vi "Process.vi"(8 "error in":errorcluster, 11 "Instrument.DAQ":refnum<class "Instrument.DAQ.lvclass">) -> (0 "error out":errorcluster, 3 "Instrument.DAQ out":refnum<class "Instrument.DAQ.lvclass">)   [LabVIEW 2019, in "Instrument.Lockin.lvlib" / "Instrument.DAQ.lvclass"]
doc: "---------------------------------------------------------------\nJKI State Machine Objects™\nhttp://jki.net/state-machine-objects/\nCopyright (C) 2005-2015, JKI <info@jki.net>\nALL RIGHTS RESERVED"
uses:
  Instrument.DAQ.lvclass
  C:/Program Files/National Instruments/LabVIEW 2019/vi.lib/JKI/JKI SMO/SMO/SMO.lvclass
  Typedefs/Status--enum.ctl
  Typedefs/DAQ.Config.AO.Range--enum.ctl
  Typedefs/DAQ.Type--enum.ctl
  Typedefs/DAQ.Config.AI.Coupling--enum.ctl
  Typedefs/DAQ.Config.AI.Range--enum.ctl
  DAQmx/typedefs/DAQmx.Status--enum.ctl
  Instrument.DAQ.lvclass/Instrument.DAQ.ctl
  Typedefs/Channel.Gain--Cluster.ctl
  Generator/typedefs/Generator.Sweep Status--enum.ctl
  Typedefs/PublicEvents--DAQ.getSweepWaveforms.ctl
  Typedefs/Results--Cluster.ctl
  <vilib>/JKI/JKI SMO/SMO/SMO.lvclass/SMO.ctl
  Typedefs/PrivateEvents--DAQ.setCalibration.ctl
  support/Simulate/Waveguide Model--Cluster.ctl
  Typedefs/PublicEvents--DAQ.getWaveforms.ctl
  Generator/typedefs/Generator.Command--enum.ctl
  6518129d-eb05-4862-8e0f-948d46b99fe2.vi
  19e91f76-1afa-420f-8f76-37c2ee2699b4.vi
  <vilib>/JKI/JKI SMO/SMO/Private/ReftoDVR--SMO.vi
  <vilib>/dlg_ctls.llb/Space Constant.vi
  <vilib>/AdvancedString/1D String Array to Delimited String.vi
  <vilib>/measure/madcrms.llb/Basic Averaged DC-RMS for N Chan.vi
  <vilib>/JKI/JKI SMO/SMO/SMO.lvclass
  <vilib>/measure/NI_MAPro.lvlib
  Instrument.Lockin/Instrument.Lockin.lvclass
  <userlib>/LevyLab/Debug/Debug.lvlib
  DAQmx/DAQmx.lvclass
  DSP/DSP.lvclass
  Waveform.Attributes/Waveform.Attributes.lvlib
  Generator/Generator.lvclass
panel:
  in  "Tab Control":enum32{"Default", "Advanced"}(tab)
  out "Sweep Chart":dbl(graph)
  out "Generator Chart":u32(graph)
  out "DSP Chart":dbl(graph)
  out "Total Chart":dbl(graph)
  out "sweep status":string
  out "Sweep Start":dbl format="%<%.3X>T"
  out "Status":T1=enum."created"
  in  "Calibrate Phase":bool
  in  "Reset Phase":bool
  out "Total (s)":dbl format="%06_6p"
  in  "Auto Phase":bool
  in  "Zero Offset":bool
  in  "Measure Offset":bool
  out "s.h.":string caption="State History"
  out "Payload":variant
  out "Generate (ms)":u32
  out "DSP (s)":dbl format="%0#6_6p"
  in  "Reset REF":bool
  out "Method":string
  out "DAQmx Status":T2
  out "start sweep":string
  out "reset":string
  in  "DAQ AO":T5(array[cluster]) {"configuration" items=["Default"=-1, "Differential"=10106, "Pseudodifferential"=12529]}
  in  "DAQ AI":T8(array[cluster]) {"configuration" items=["default"=-1, "Differential"=10106, "Pseudodifferential"=12529]; "Coupling" items=[""=0, "AC"=10045, "DC"=10050, "GND"=10066]}
  # "For instructions on how to use the JKI State Machine Objects, examples and video tutorials, visit:\nhttp://jki.net/state-machine-objects/\n\nJKI State Machine Objects™\nhttp://jki.net/state-machine-objects/\nCopyright (C) 2005-2015, JKI <info@jki.net>\nALL RIGHTS RESERVED"
  # "DAQ"
  # "State"
  # "Messages"
  # "Sweep"
  # "Controls"
  # "Timing"
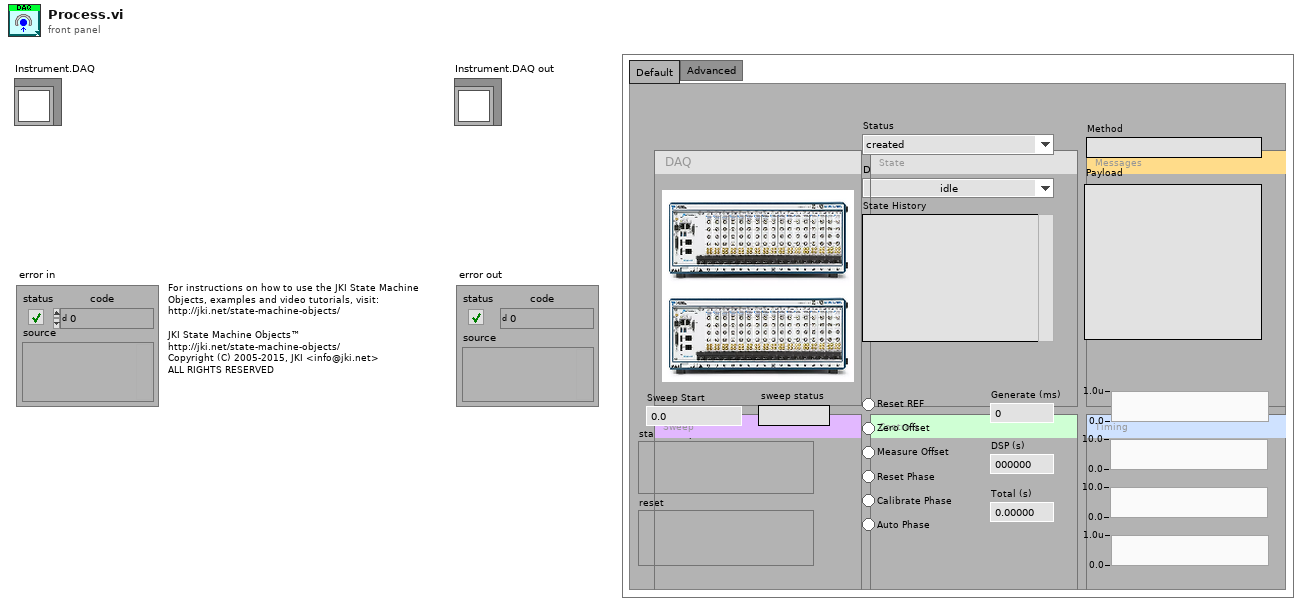
[diagram p1: front panel]
types:
  T1 = typedef "Instrument.Lockin.lvlib/Instrument.DAQ.lvclass/Status--enum.ctl" = enum16{"idle", "created", "started", "stopped", "sweeping"}
  T2 = typedef "DAQmx.lvclass/DAQmx.Status--enum.ctl" = enum16{"idle", "calibrating", "configuring", "creating", "created", "starting", "started", "stopping", "stopped", "clearing", "error"}
  T3 = typedef "Instrument.Lockin.lvlib/Instrument.DAQ.lvclass/DAQ.Config.AO.Range--enum.ctl" = enum16{"±0.1", "±1.0", "±3.5", "±10.0", ""}
  T4 = typedef "Instrument.Lockin.lvlib/Instrument.DAQ.lvclass/DAQ.Type--enum.ctl" = enum16{"None", "USB-4431", "PXI-446x"}
  T5 = cluster{"Channel":tag, "Range":T3, "configuration":i32, "Type":T4}[]
  T6 = typedef "Instrument.Lockin.lvlib/Instrument.DAQ.lvclass/DAQ.Config.AI.Coupling--enum.ctl" = u16
  T7 = typedef "Instrument.Lockin.lvlib/Instrument.DAQ.lvclass/DAQ.Config.AI.Range--enum.ctl" = enum16{"±0.316", "±1.00", "±3.16", "±10.0", "±31.6", "±42.4", ""}
  T8 = cluster{"Channel":tag, "Coupling":T6, "Range":T7, "configuration":i32, "Type":T4}[]
  T9 = typedef "Instrument.Lockin.lvlib/Instrument.DAQ.lvclass/Channel.Gain--Cluster.ctl" = cluster{"Channel":string, "Gain":dbl}
  T10 = enum32{"invalid app kind", "Development System", "Run Time System", "Student Edition", "Embedded LabVIEW", "Evaluation", "Custom"}
  T11 = typedef "Instrument.Lockin.lvlib/Instrument.DAQ.lvclass/PublicEvents--DAQ.getSweepWaveforms.ctl" = cluster{"AO":waveform(dbl)[], "AI":waveform(dbl)[], "X":waveform(dbl)[], "Y":waveform(dbl)[]}
  T12 = enum32{"Invalid", "Standard", "Closed", "Hidden", "Minimized", "Maximized"}
  T13 = typedef "Generator.lvclass/Generator.Sweep Status--enum.ctl" = enum16{"idle", "initializing", "waiting", "sweeping", "stopping"}
  T14 = typedef "Instrument.Lockin.lvlib/Instrument.DAQ.lvclass/PrivateEvents--DAQ.setCalibration.ctl" = enum16{"Check", "Calibrate"}
  T15 = typedef "Instrument.Lockin.lvlib/Instrument.DAQ.lvclass/Waveguide Model--Cluster.ctl" = cluster{"I+":i32, "I-":i32, "V+":i32, "V-":i32, "Vsg":i32}
  T16 = typedef "Instrument.Lockin.lvlib/Instrument.DAQ.lvclass/PublicEvents--DAQ.getWaveforms.ctl" = cluster{"AO":waveform(dbl)[], "AI":waveform(dbl)[], "REF_X":waveform(dbl)[], "REF_Y":waveform(dbl)[], "X":waveform(dbl)[], "Y":waveform(dbl)[]}
  T17 = typedef "Generator.lvclass/Generator.Command--enum.ctl" = enum16{"start", "stop", "start sweep", "stop sweep"}
  T18 = typedef "Instrument.Lockin.lvlib/Instrument.DAQ.lvclass/Results--Cluster.ctl" = cluster{"Time Stamp":timestamp, "Results (Dictionary)":cluster{"key":string, "value":dbl[]}[]}
  T19 = cluster{"Core":cluster{"Current VI Reference":refnum<vi>, "Close Panel on Exit?":bool, "Last Error":cluster{"error":errorcluster, "previous state":string, "remaining states":string}, "Shutdown?":bool}, "SMO":refnum<class "Instrument.DAQ.lvclass">, "DAQ Status":T1, "DAQmx Status":T2, "Sweep Status":T13, "Results":T18, "SweepWaveforms":T11, "Measure Offset":bool, "Saved Amplitudes":dbl[]}
  T20 = typedef "Instrument.Lockin.lvlib/Instrument.DAQ.lvclass/DAQ.Config.AO--Cluster--Array.ctl" = cluster{"Channels":tag, "Range":T3, "terminal configuration":T21, "Type":T4}[]
  T21 = typedef "Instrument.Lockin.lvlib/Instrument.DAQ.lvclass/DAQ.TerminalConfiguration--ring.ctl" = i32
  T22 = cluster{"Channels":tag, "Range":T3, "terminal configuration":T21, "Type":T4}
  T23 = typedef "Instrument.Lockin.lvlib/Instrument.DAQ.lvclass/DAQ.Config.AI--Cluster--Array.ctl" = cluster{"Channels":tag, "Coupling":T6, "Range":T7, "terminal configuration":T21, "Type":T4}[]
  T24 = typedef "Instrument.Lockin.lvlib/Instrument.DAQ.lvclass/Simulation Mode--enum.ctl" = enum16{"AI = HW simulated", "AI = noise*AO", "AI = waveguide"}
  T25 = cluster{"AI Configuration":T23, "Simulation mode":T24}
  T26 = cluster{"Channels":tag, "Coupling":T6, "Range":T7, "terminal configuration":T21, "Type":T4}
  T27 = typedef "Instrument.Lockin.lvlib/Instrument.DAQ.lvclass/AO.Channel--Cluster--Array.ctl" = T28[]
  T28 = typedef "Instrument.Lockin.lvlib/Instrument.DAQ.lvclass/AO.Channel--Cluster.ctl" = cluster{"Enable?":bool, "Channel":i32, "Amplitude":dbl, "Offset":dbl, "Frequency":dbl, "Phase":dbl, "Function":T29, "Sweeping?":bool, "Limit AC":bool, "Limit DC?":bool, "Duty Cycle":bool}
  T29 = typedef "Instrument.Lockin.lvlib/Instrument.DAQ.lvclass/AO.Channel.Function--Enum.ctl" = enum16{"sine", "square", "triangle", "saw"}
  T30 = typedef "Instrument.Lockin.lvlib/Instrument.DAQ.lvclass/AI.Channel--Cluster--Array.ctl" = T31[]
  T31 = typedef "Instrument.Lockin.lvlib/Instrument.DAQ.lvclass/AI.Channel--Cluster.ctl" = cluster{"Enable?":bool, "Channel":i32, "References":u16[], "reference index":i32}
  T32 = typedef "Instrument.Lockin.lvlib/Instrument.DAQ.lvclass/REF.Channel--Cluster--Array.ctl" = T33[]
  T33 = typedef "Instrument.Lockin.lvlib/Instrument.DAQ.lvclass/REF.Channel--Cluster.ctl" = cluster{"Enable?":bool, "Channel":i32, "Frequency":dbl, "Phase":dbl, "TC":dbl, "Roll-Off":i32}
  T34 = typedef "Instrument.Lockin.lvlib/Instrument.DAQ.lvclass/DAQ.Sampling--Cluster.ctl" = cluster{"Sampling":T35, "sample mode":i32, "Fs Mode":T36, "Fs Multiplier":dbl, "Refresh Rate (Hz)":dbl, "Decimation.PreDSP":i32, "Decimation.PostDSP":i32, "Fs.Output":dbl}
  T35 = typedef "Instrument.Lockin.lvlib/Instrument.DAQ.lvclass/DAQ.Sampling.Sampling--Cluster.ctl" = cluster{"Fs":dbl, "#s":i32}
  T36 = typedef "Instrument.Lockin.lvlib/Instrument.DAQ.lvclass/DAQ.Sampling.Fs Mode--enum.ctl" = enum16{"Manual", "Auto Fs", "Max Fs"}
  T37 = typedef "Instrument.Lockin.lvlib/Instrument.DAQ.lvclass/Sweep.Configuration--Cluster.ctl" = cluster{"sweepTime":dbl, "initialWaitTime":dbl, "returnToStart":bool, "sweepChannels":T38}
  T38 = typedef "Instrument.Lockin.lvlib/Instrument.DAQ.lvclass/Sweep.Channel--Cluster--Array.ctl" = T39[]
  T39 = typedef "Instrument.Lockin.lvlib/Instrument.DAQ.lvclass/Sweep.Channel--Cluster.ctl" = cluster{"Enable?":bool, "Channel":u16, "Start":dbl, "End":dbl, "Pattern":T40, "Table":dbl[]}
  T40 = typedef "Instrument.Lockin.lvlib/Instrument.DAQ.lvclass/Sweep.Pattern--Enum.ctl" = enum16{"Ramp /", "Ramp /\\", "Smooth Ramp _/", "Smooth Ramp _/\\_", "Table"}
  T41 = typedef "Instrument.Lockin.lvlib/Instrument.DAQ.lvclass/PrivateEvents--DAQ.measureOffset.ctl" = bool
  T42 = typedef "Instrument.Lockin.lvlib/Instrument.DAQ.lvclass/PrivateEvents--DAQ.zeroPhase.ctl" = bool
  T43 = typedef "Instrument.Lockin.lvlib/Instrument.DAQ.lvclass/Configuration.Prefilter--Cluster.ctl" = cluster{"60 Hz":bool, "Low Pass":bool, "Low Pass Cutoff (Hz)":dbl}
  T44 = typedef "Instrument.Lockin.lvlib/Instrument.DAQ.lvclass/Configuration.AmplitudeLimit--Cluster.ctl" = cluster{"Limit?":bool, "Limit (V)":dbl}
  T45 = typedef "Instrument.Lockin.lvlib/Instrument.DAQ.lvclass/Configuration.DCLimit--Cluster.ctl" = cluster{"Limit?":bool, "Limit (V)":dbl}
  T46 = typedef "Instrument.Lockin.lvlib/Instrument.DAQ.lvclass/Configuration.DutyCycle--Cluster.ctl" = cluster{"Option?":bool, "Duty Cycle (%)":dbl}
  T47 = typedef "Instrument.Lockin.lvlib/Instrument.DAQ.lvclass/Configuration.LinkFrequencies--Cluster.ctl" = cluster{"Link?":bool, "Frequency (Hz)":dbl}
  T48 = typedef "Instrument.Lockin.lvlib/Instrument.DAQ.lvclass/State--enum.ctl" = enum16{"start", "stop", "reset", "start sweep", "stop sweep"}
  T49 = typedef "Instrument.Lockin.lvlib/Instrument.DAQ.lvclass/PrivateEvents--DAQ.showUI.ctl" = bool
  T50 = typedef "DAQmx.lvclass/DeviceInfo--Cluster.ctl" = cluster{"DeviceName":string, "DevIsSimulated":bool, "DeviceSerialNumber":string, "ProductType":string, "ProductCategory":i32, "ProductNumber":u32, "ChassisNumber":u32, "SlotNumber":u32, "ChassisName":string, "ChassisSerialNumber":string, "DevTemp":dbl, "SelfCal.LastDate/Time":string, "SelfCal.LastTemp":dbl, "calibration due?":bool}
  T51 = cluster{"Active Device":string, "SelfCal.LastDate/Time":string, "SelfCal.LastTemp":dbl, "DevTemp":dbl, "calibration due?":bool}[]
  T52 = typedef "Instrument.Lockin.lvlib/Instrument.DAQ.lvclass/DAQ.Calibration--Cluster.ctl" = cluster{"Active Device":string, "SelfCal.LastDate/Time":dbl, "SelfCal.LastTemp":dbl, "DevTemp":dbl, "calibration due?":bool}
  T53 = typedef "DAQmx.lvclass/DAQ.Config.AO--Cluster--Array.ctl" = T54[]
  T54 = typedef "DAQmx.lvclass/DAQ.Config.AO--Cluster.ctl" = cluster{"Channels":tag, "Range":T55, "output terminal configuration":i32, "Type":T56}
  T55 = typedef "DAQmx.lvclass/DAQ.Config.AO.Range--enum.ctl" = enum16{"±0.1", "±1.0", "±3.5", "±10.0", ""}
  T56 = typedef "DAQmx.lvclass/DAQ.Config.Device Type--enum.ctl" = enum16{"None", "USB-4431", "PXI-446x"}
  T57 = typedef "DAQmx.lvclass/DAQ.Config.AI--Cluster--Array.ctl" = T58[]
  T58 = typedef "DAQmx.lvclass/DAQ.Config.AI--Cluster.ctl" = cluster{"Channels":tag, "Coupling":T59, "Range":T60, "input terminal configuration":i32, "Type":T56}
  T59 = typedef "DAQmx.lvclass/DAQ.Config.AI.Coupling--enum.ctl" = u16
  T60 = typedef "DAQmx.lvclass/DAQ.Config.AI.Range--enum.ctl" = enum16{"±0.316", "±1.00", "±3.16", "±10.0", "±31.6", "±42.4", ""}
  T61 = typedef "Generator.lvclass/AO.Channel--Cluster--Array.ctl" = T62[]
  T62 = typedef "Generator.lvclass/AO.Channel--Cluster.ctl" = cluster{"Enable?":bool, "Channel":i32, "Amplitude":dbl, "Offset":dbl, "Frequency":dbl, "Phase":dbl, "Function":T63, "Sweeping?":bool, "Limit AC?":bool, "Limit DC?":bool, "Duty Cycle?":bool, "Duty Cycle":dbl}
  T63 = typedef "Generator.lvclass/AO.Channel.Function--Enum.ctl" = enum16{"sine", "square", "triangle", "saw"}
  T64 = cluster{"Current VI Reference":refnum<vi>, "Close Panel on Exit?":bool, "Last Error":cluster{"error":errorcluster, "previous state":string, "remaining states":string}, "Shutdown?":bool}
  T65 = typedef "Instrument.Lockin.lvlib/Instrument.DAQ.lvclass/DeviceInfo--Cluster.ctl" = cluster{"DeviceName":string, "DevIsSimulated":bool, "DeviceSerialNumber":string, "ProductType":string, "ProductCategory":i32, "ProductNumber":u32, "ChassisNumber":u32, "SlotNumber":u32, "ChassisName":string, "ChassisSerialNumber":string, "DevTemp":dbl, "SelfCal.LastDate/Time":string, "SelfCal.LastTemp":dbl, "calibration due?":bool}
  T66 = typedef "Instrument.Lockin.lvlib/Instrument.DAQ.lvclass/DAQ.Calibration--Cluster--Array.ctl" = T52[]
  T67 = typedef "Instrument.Lockin.lvlib/Instrument.DAQ.lvclass/DAQ.Configuration--Cluster--Array.ctl" = T68[]
  T68 = typedef "Instrument.Lockin.lvlib/Instrument.DAQ.lvclass/DAQ.Configuration--Cluster.ctl" = cluster{"Device":string, "Lockin.AO":string, "AO.Ch":string, "AO.Range":T3, "AO terminal config":T21, "Lockin.AI":string, "AI.Ch":string, "AI.Range":T7, "AI.Coupling":T6, "AI terminal config":T21}
  T69 = typedef "Instrument.Lockin.lvlib/Instrument.DAQ.lvclass/Channel.Gain--Cluster--Array.ctl" = T9[]
  T70 = typedef "Debug.lvlib/Attribute.Debug.lvclass/DebugBehavior.ctl" = enum16{"Normal", "Debug"}
  T71 = typedef "SMO.lvclass/Protected Events.ctl" = cluster{"StopProcesses":refnum<user-event>, "AbortProcesses":refnum<user-event>, "Config Changed":refnum<user-event>, "Dependency":refnum<user-event>}
  T72 = typedef "Instrument.Lockin.lvlib/Instrument.DAQ.lvclass/PrivateEvents--Cluster.ctl" = cluster{"setAOconfig":refnum<user-event>, "setAIconfig":refnum<user-event>, "setAO":refnum<user-event>, "setREF":refnum<user-event>, "setSampling":refnum<user-event>, "setState":refnum<user-event>, "setInputGain":refnum<user-event>, "setOutputGain":refnum<user-event>, "setSweep":refnum<user-event>, "measureOffset":refnum<user-event>, "zeroOffset":refnum<user-event>, "setPreFilter":refnum<user-event>, "autoConfigureDAQ":refnum<user-event>, "setCalibration":refnum<user-event>, "setAI":refnum<user-event>, "zeroPhase":refnum<user-event>, "setAmplitudeLimit":refnum<user-event>, "setLinkFrequencies":refnum<user-event>, "showUI":refnum<user-event>, "setInputOffset":refnum<user-event>, "setDCLimit":refnum<user-event>, "setDutyCycle":refnum<user-event>}
  T73 = typedef "DAQmx.lvclass/PublicEvents--Cluster.ctl" = cluster{"Status":refnum<user-event>, "Devices":refnum<user-event>, "Calibration":refnum<user-event>, "Sampling":refnum<user-event>, "AOconfig":refnum<user-event>, "AIconfig":refnum<user-event>, "Waveforms":refnum<user-event>}
  T74 = typedef "Generator.lvclass/PublicEvents--Cluster.ctl" = cluster{"Status":refnum<user-event>, "SweepStatus":refnum<user-event>, "AOChannels":refnum<user-event>, "Waveforms":refnum<user-event>}
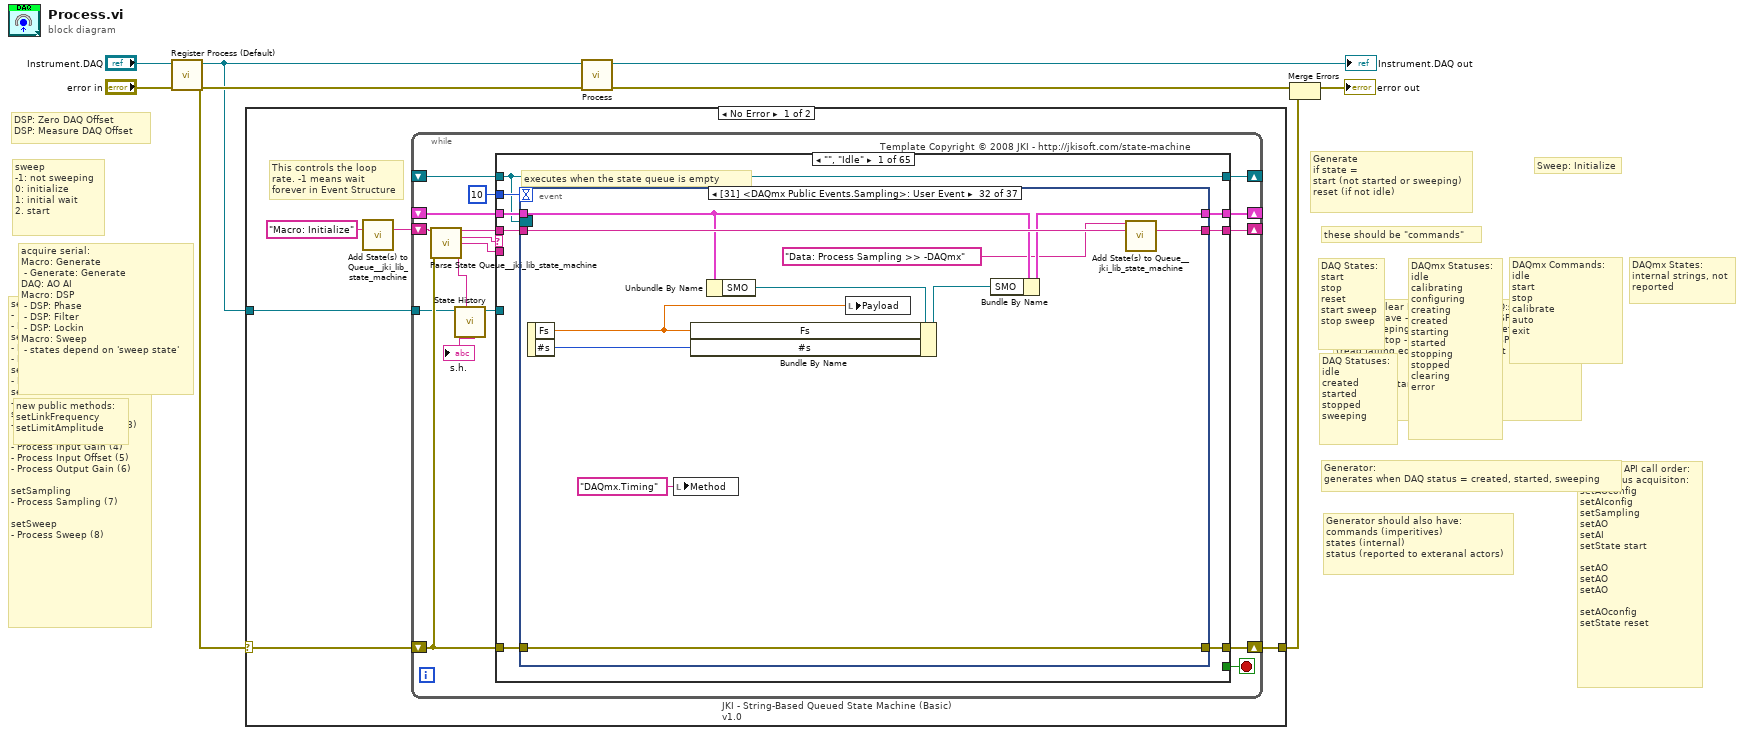
[diagram p0: block diagram]
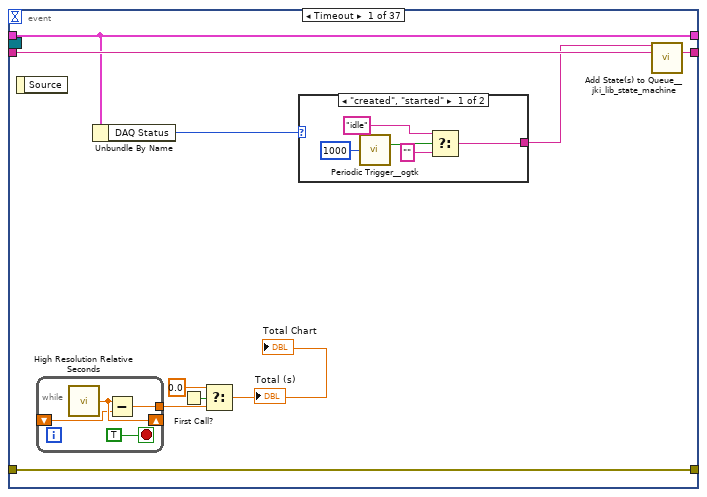
[diagram p2: hidden frame]
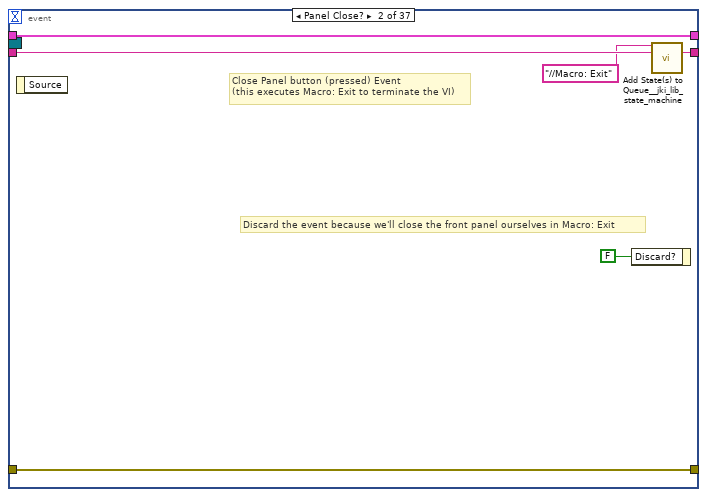
[diagram p4: hidden frame]
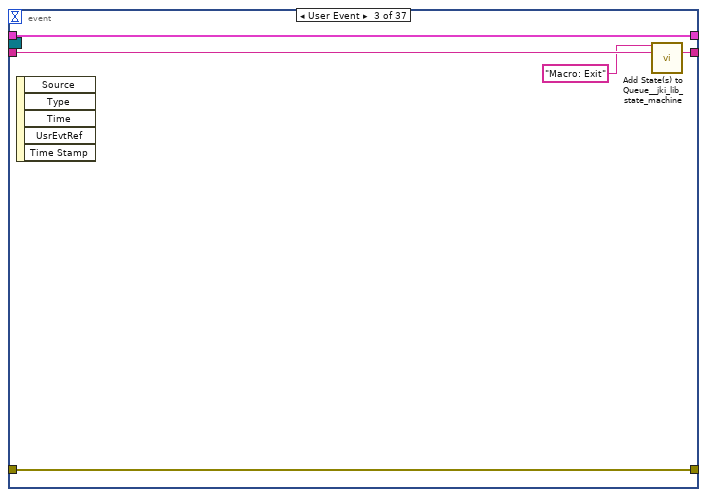
[diagram p5: hidden frame]
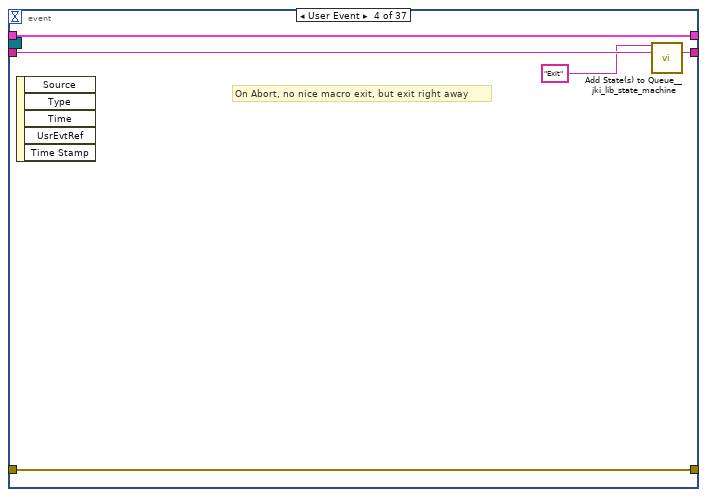
[diagram p6: hidden frame]
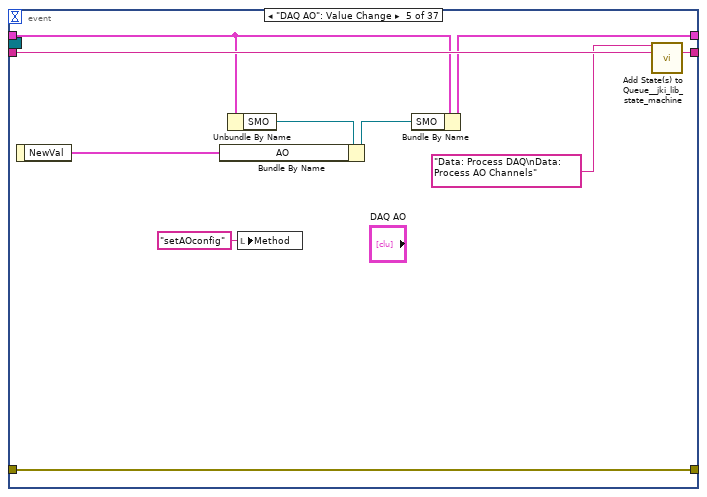
[diagram p7: hidden frame]
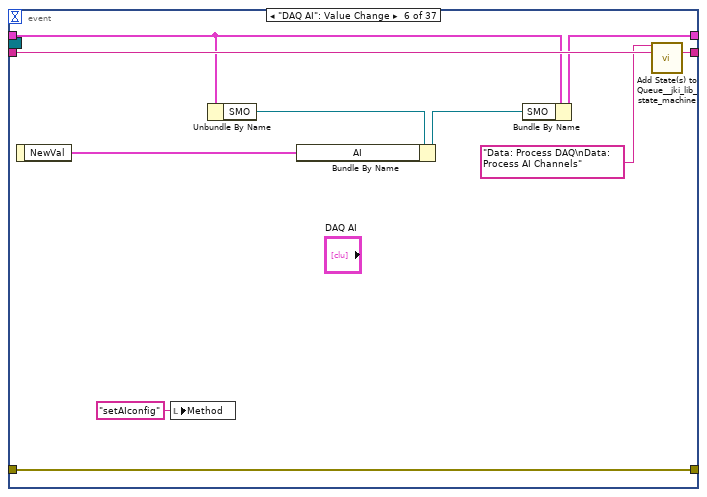
[diagram p8: hidden frame]
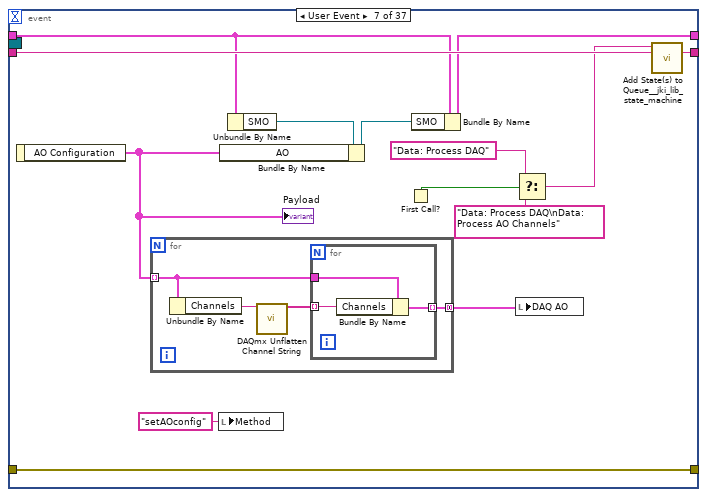
[diagram p9: hidden frame]
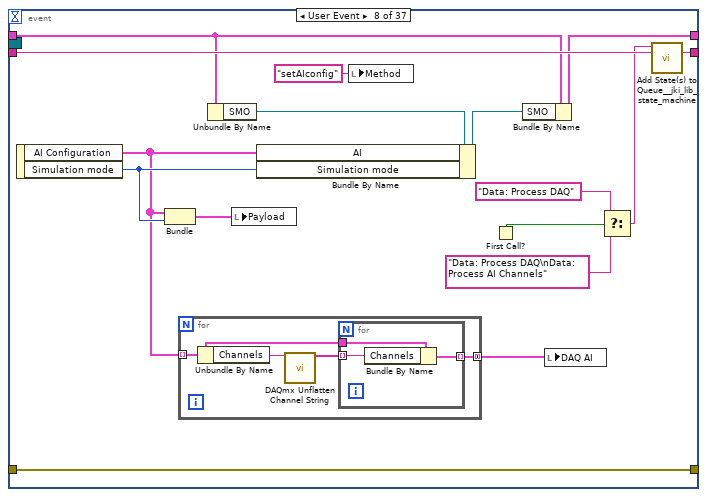
[diagram p10: hidden frame]
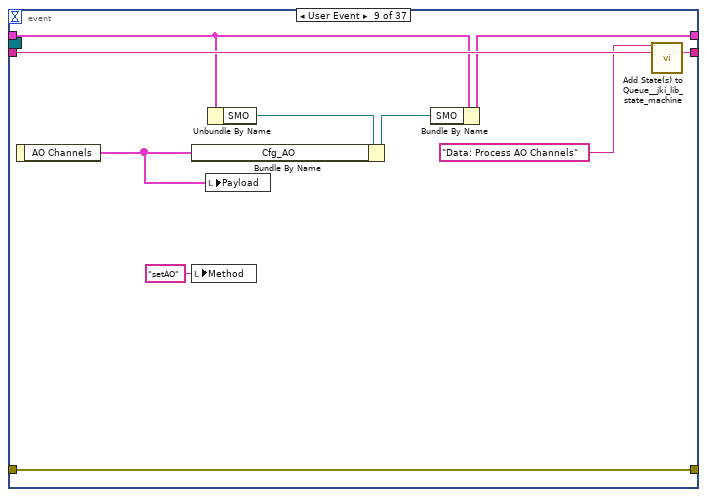
[diagram p11: hidden frame]
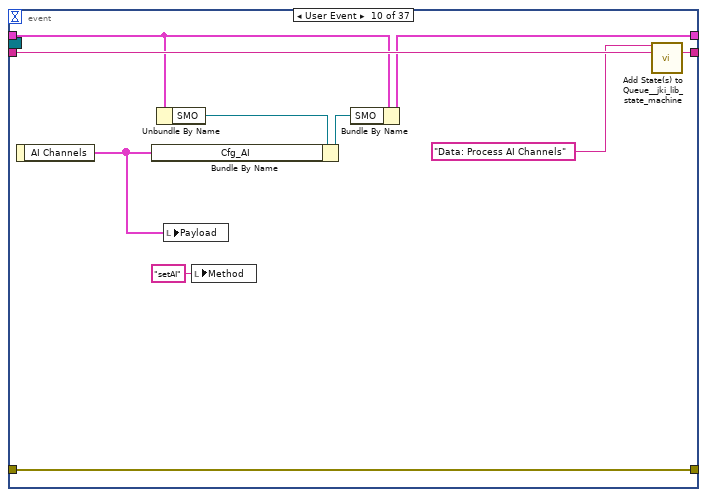
[diagram p12: hidden frame]
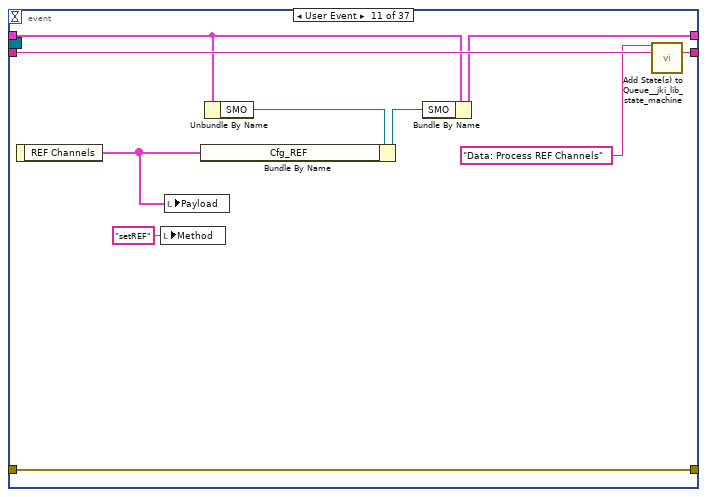
[diagram p13: hidden frame]
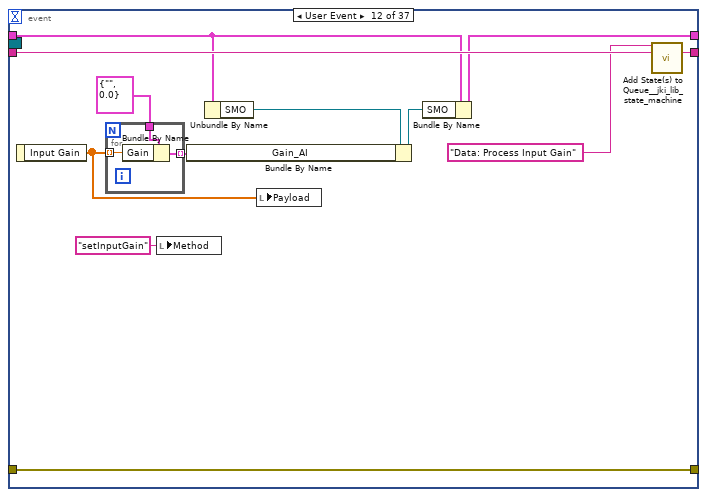
[diagram p14: hidden frame]
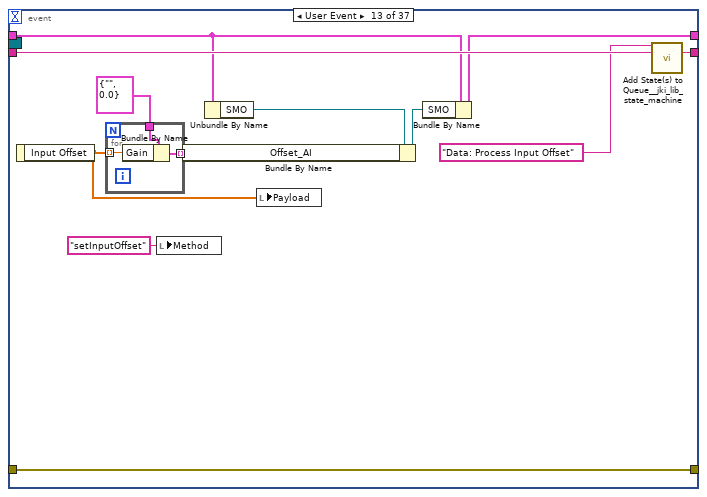
[diagram p15: hidden frame]
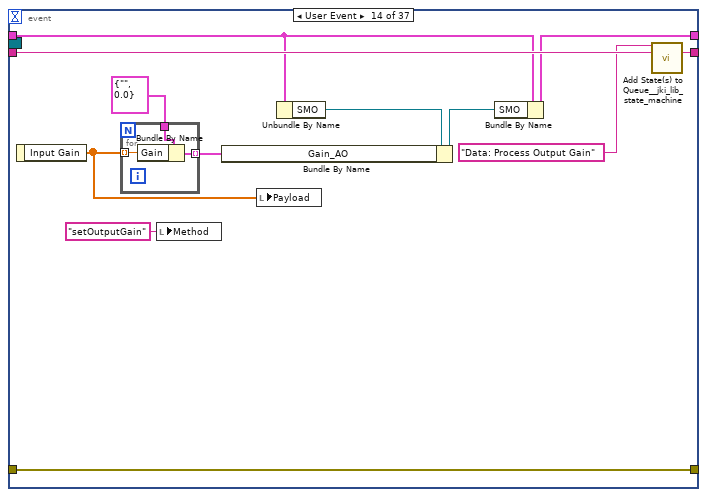
[diagram p16: hidden frame]
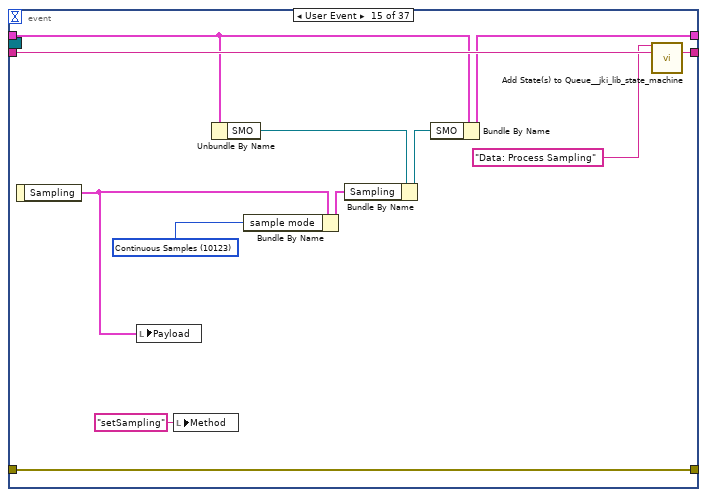
[diagram p17: hidden frame]
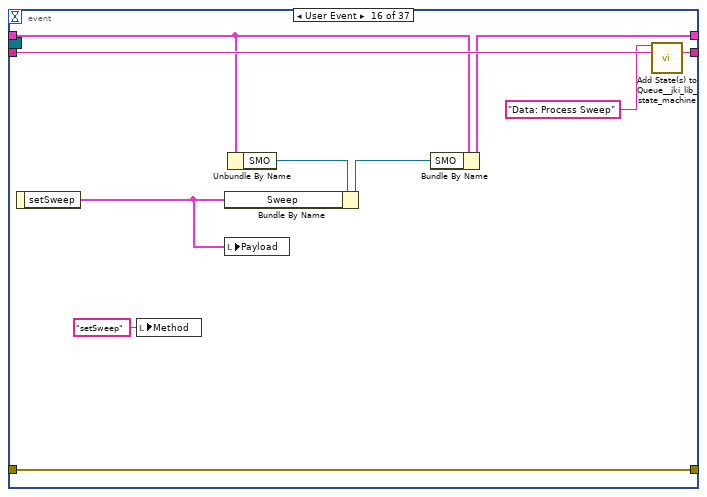
[diagram p18: hidden frame]
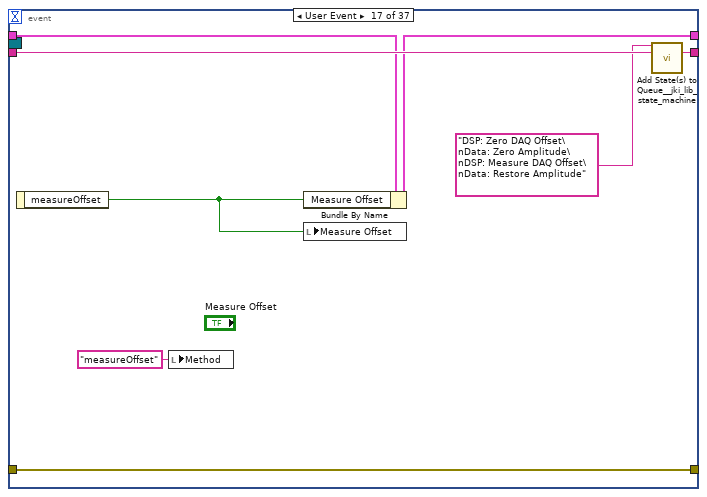
[diagram p19: hidden frame]
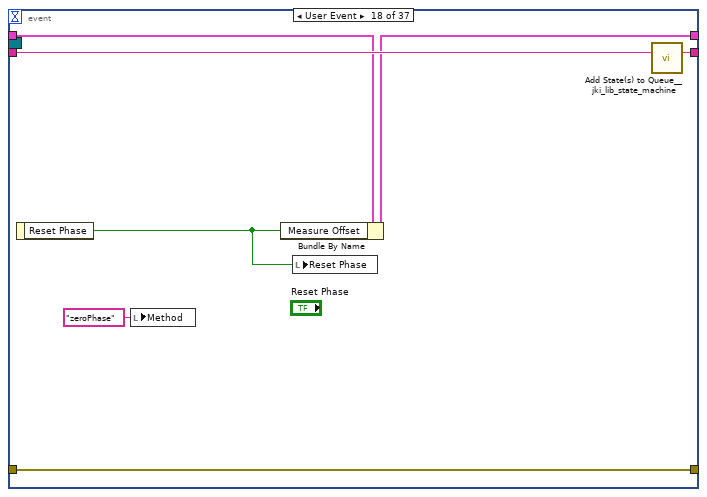
[diagram p20: hidden frame]
diagram:
  # "Sweep: Initialize"
  # "- Sweep: Clear Data - called by DAQ:setState\n- Sweep: Save - called by Macro: DSP\n(read sweeping attribute from waveform)\n- Sweep: Stop - called by Macro: DSP\n(read falling edge sweeping --> not sweeping)\n\n\nGenerator: Start, Stop"
  # "example API call order:\ncontinuous acquisiton:\nsetAOconfig\nsetAIconfig\nsetSampling\nsetAO\nsetAI\nsetState start\n\nsetAO\nsetAO\nsetAO\n\nsetAOconfig\nsetState reset"
  # "Generator should also have:\ncommands (imperitives)\nstates (internal)\nstatus (reported to exteranal actors)"
  # "these should be \"commands\""
  # "DAQmx States:\ninternal strings, not\nreported"
  # "DAQmx Commands:\nidle\nstart\nstop\ncalibrate\nauto\nexit"
  # "Generator:\ngenerates when DAQ status = created, started, sweeping"
  # "DAQmx Statuses:\nidle\ncalibrating\nconfiguring\ncreating\ncreated\nstarting\nstarted\nstopping\nstopped\nclearing\nerror"
  # "DAQ Statuses:\nidle\ncreated\nstarted\nstopped\nsweeping"
  # "DAQ States:\nstart\nstop\nreset\nstart sweep\nstop sweep"
  # "Generate\nif state = \nstart (not started or sweeping)\nreset (if not idle)"
  # "setAOconfig:\n-\t Process DAQ (0)\n- Process AO Channels (1)\nsetAOconfig\n- Process DAQ\n- Process AI Channels (2)\nsetAO\n- Process AO Channels\nsetAI\n- Process AI Channels\nsetREF\n- Process REF Channels (3)\n\n- Process Input Gain (4)\n- Process Input Offset (5)\n- Process Output Gain (6)\n\nsetSampling\n- Process Sampling (7)\n\nsetSweep\n- Process Sweep (8)"
  # "acquire serial:\nMacro: Generate\n - Generate: Generate\nDAQ: AO AI\nMacro: DSP\n - DSP: Phase\n - DSP: Filter\n - DSP: Lockin\nMacro: Sweep\n - states depend on 'sweep state'"
  # "sweep\n-1: not sweeping\n0: initialize\n1: initial wait\n2. start"
  # "DSP: Zero DAQ Offset\nDSP: Measure DAQ Offset"
  # "new public methods:\nsetLinkFrequency\nsetLimitAmplitude"
  n1 = call <vilib>:"Register Process (Default).vi"("error in (no error)"="error in", "SMO"="Instrument.DAQ") -> ("error out"=w5:errorcluster, "SelfRef"=w4:refnum<class "Instrument.DAQ.lvclass">)  [unwired: 8 in]
  n2 = case shown="No Error" w5 {
    selector: w5 -> [w13 w1355]
    tunnel: w4 -> [w9 _]
    tunnel: [w12 w1355] -> w1
    frame No Error {
      # "This controls the loop rate. -1 means wait forever in Event Structure"
      n3 = call <vilib>:"Add State(s) to Queue__jki_lib_state_machine.vi"("State(s) in (\"\")"="Macro: Initialize") -> ("States Out"=w11:string)  [unwired: 14 in]
      n4 = while "JKI - String-Based Queued State Machine (Basic) v1.0" {
        shift-right: [w24] -> _
        shift-left: _ -> [w20]
        shift-right: [w19] -> w12
        shift-left: w13 -> [w23]
        shift-right: [w26] -> _
        shift-left: w11 -> [w27]
        tunnel: w9 -> [w14]
        shift-right: [w22] -> _
        shift-left: _ -> [w21]
        stop <- w25 stop-if-true
        # "Template Copyright © 2008 JKI - http://jkisoft.com/state-machine"
        n5 = call <vilib>:"Parse State Queue__jki_lib_state_machine.vi"("State Queue"=w27, "Error In (no error)"=w23) -> ("Remaining States"=w29:string, "Current State"=w17:string, "Arguments"=w28:string)  [unwired: 11 in]
        n6 = call <userlib>:"State History.vi"("Current State"=w17, "SMO"=w14) -> ("SMO"=w15:refnum<class "Instrument.DAQ.lvclass">, "History"=→"s.h.":string)  [unwired: 8 in]
        n7 = case shown="\"\", \"Idle\"" w17 {
          selector: w17 -> [_ _ w473 _ _ _ _ _ _ _ _ _ _ _ _ _ _ _ _ _ _ _ _ _ _ _ _ _ _ w867 _ _ _ _ _ _ _ _ _ _ _ _ _ _ _ _ _ _ _ _ _ _ _ _ _ _ _ _ _ _ _ _ _ _ _]
          tunnel: w29 -> [w37 w471 w477 w496 w498 w515 w520 w535 w546 w567 w577 w593 w622 w643 w668 w688 w700 w712 w724 w741 w750 w765 w775 w787 w811 w832 w848 w853 w862 w878 w885 w901 w933 w942 w957 w976 w1010 w1017 w1034 w1064 w1069 w1080 w1085 w1105 w1111 w1116 w1125 w1134 w1147 w1164 w1169 w1179 w1199 w1229 w1246 w1264 w1284 w1301 w1306 w1313 w1318 w1327 w1336 w1345 w1354]
          tunnel: w28 -> [_ _ _ _ _ _ _ _ _ _ _ w578 w615 _ _ _ _ _ _ _ _ _ _ _ w789 _ _ _ _ w863 w879 w895 _ _ _ _ _ _ _ _ _ _ _ _ _ _ _ _ w1136 _ _ _ _ _ _ _ _ _ _ _ _ _ _ _ _]
          tunnel: w20 -> [w35 w468 w475 w487 w507 w511 w517 _ w540 w562 w568 w589 w618 w639 w664 w684 w695 w708 w719 w737 w746 w759 w771 w783 w807 w826 w842 w850 w860 w875 w883 w897 w930 w938 w945 w965 w994 w1012 w1028 w1054 w1066 w1077 w1082 w1103 w1109 w1114 w1120 w1131 w1144 w1161 w1167 w1172 w1195 w1226 w1243 w1260 w1281 w1297 w1304 w1307 w1316 w1324 w1333 w1342 w1351]
          tunnel: w23 -> [w33 w469 w478 w493 w499 _ w518 w528 w541 w559 w570 w582 w608 w636 w662 w683 w691 w702 w714 w735 w742 w757 w769 w781 w798 w828 w845 w851 w856 w876 w881 w899 w931 w940 w943 w974 w1008 w1015 w1033 w1049 w1067 w1072 w1083 w1088 w1108 w1112 w1121 w1126 w1141 w1157 w1165 w1174 w1192 w1223 w1232 w1261 w1266 w1294 w1302 w1310 w1314 w1320 w1329 w1338 w1347]
          tunnel: [w36 w470 w476 w495 w502 w514 w519 w534 w545 w566 w576 w592 w621 w642 w667 w687 w699 w711 w723 w740 w749 w764 w774 w786 w810 w831 w847 w852 w861 w877 w884 w900 w932 w941 w956 w975 w1009 w1016 w1031 w1063 w1068 w1079 w1084 w1104 w1110 w1115 w1124 w1133 w1146 w1163 w1168 w1178 w1198 w1228 w1245 w1263 w1283 w1300 w1305 w1312 w1317 w1326 w1335 w1344 w1353] -> w26
          tunnel: [_ _ _ _ _ TRUE _ _ _ _ _ _ _ _ _ _ _ _ _ _ _ _ _ _ _ _ _ _ _ _ _ _ _ _ _ _ _ _ _ _ _ _ _ _ _ _ _ _ _ _ _ _ _ _ _ _ _ _ _ _ _ _ _ _ _] -> w25
          tunnel: [w32 w468 w475 w494 w506 w511 w517 w532 w542 w563 w569 w590 w619 w640 w665 w685 w696 w709 w720 w738 w746 w760 w772 w784 w808 w827 w842 w850 w860 w875 w883 w897 w930 w938 w947 w966 w995 w1012 w1028 w1054 w1066 w1077 w1082 w1103 w1109 w1114 w1119 w1130 w1143 w1160 w1167 w1173 w1194 w1225 w1242 w1260 w1280 w1296 w1304 w1307 w1316 w1324 w1333 w1342 w1351] -> w24
          tunnel: 10 ("to") -> [w31 _ _ _ _ _ _ _ _ _ _ _ _ _ _ _ _ _ _ _ _ _ _ _ _ _ _ _ _ _ _ _ _ _ _ _ _ _ _ _ _ _ _ _ _ _ _ _ _ _ _ _ _ _ _ _ _ _ _ _ _ _ _ _ _]
          tunnel: w15 -> [_ _ _ _ _ _ _ w527 _ _ _ _ _ _ _ _ _ _ _ _ _ _ _ _ _ _ _ _ _ _ _ _ _ _ _ _ _ _ _ _ _ _ _ _ _ _ _ _ _ _ _ _ _ _ _ _ _ _ _ _ _ _ _ _ _]
          tunnel: [w30 w467 w472 w484 w509 w512 w516 w533 w544 w565 w575 w591 w620 w641 w666 w686 w698 w710 w722 w739 w748 w763 w773 w785 w809 w830 w843 w849 w859 w874 w882 w894 w929 w939 w955 w973 w1003 w1014 w1032 w1062 w1065 w1078 w1081 w1097 w1106 w1113 w1123 w1132 w1145 w1162 w1166 w1177 w1197 w1227 w1244 w1262 w1282 w1299 w1303 w1311 w1315 w1325 w1334 w1343 w1352] -> w22
          tunnel: w21 -> [w30 w467 w472 w484 w509 w512 w516 w533 w544 w565 w575 w591 w620 w641 w666 w686 w698 w710 w722 w739 w748 w763 w773 w785 w809 w830 w843 w849 w859 w874 w882 w894 w929 w939 w955 w973 w1003 w1014 w1032 w1062 w1065 w1078 w1081 _ w1106 w1113 w1123 w1132 w1145 w1162 w1166 w1177 w1197 w1227 w1244 w1262 w1282 w1299 w1303 w1311 w1315 w1325 w1334 w1343 w1352]
          tunnel: [w34 w469 w479 w493 errorcluster {"status"=FALSE, "code"=0, "source"=""} ("No error") w510 w518 w530 w537 w560 w571 w579 w604 w631 w655 w669 w690 w706 w715 w734 w743 w758 w768 w779 w797 w829 w844 w851 w857 w876 w880 w898 w931 w940 w944 w974 w1008 w1015 w1033 w1050 w1067 w1071 w1083 w1101 w1108 w1112 w1117 w1127 w1140 w1156 w1165 w1175 w1185 w1213 w1237 w1261 w1267 w1288 w1302 w1310 w1314 w1321 w1330 w1339 w1348] -> w19
          frame "", "Idle" {
            # "executes when the state queue is empty"
            n8 = event shown="[31] <DAQmx Public Events.Sampling>: User Event" {
              selector: w30 -> [_ _ _ _ _ _ _ _ _ _ _ _ _ _ _ _ _ _ _ _ _ _ _ _ _ _ _ _ _ _ _ _ _ _ _ _ _]
              dyn-events: _ -> [_ _ _ _ _ _ _ _ _ _ _ _ _ _ _ _ _ _ _ _ _ _ _ _ _ _ _ _ _ _ _ _ _ _ _ _ _]
              timeout: w31 -> [_ _ _ _ _ _ _ _ _ _ _ _ _ _ _ _ _ _ _ _ _ _ _ _ _ _ _ _ _ _ _ _ _ _ _ _ _]
              tunnel: w37 -> [w42 w63 w68 w73 w83 w93 w107 w130 w147 w157 w167 w179 w194 w209 w224 w234 w242 w249 w255 w265 w275 w285 w295 w305 w312 w320 w342 w353 w360 w370 w381 w392 w402 w412 w430 w445 w459]
              tunnel: [w47 w62 w67 w72 w82 w92 w106 w129 w146 w156 w166 w178 w193 w208 w223 w233 w241 w248 w254 w264 w274 w284 w294 w304 w311 w319 w341 w352 w361 w371 w382 w393 w403 w413 w431 w444 w460] -> w36
              tunnel: w35 -> [w41 w60 w65 w70 w79 w89 w103 w126 w143 w153 w163 w175 w190 w205 w221 w230 w238 w246 w252 w260 w270 w280 w290 w300 w309 w314 w337 w349 w358 w366 w377 w387 w395 w406 w426 w440 w462]
              tunnel: [w46 w61 w66 w71 w76 w86 w100 w121 w142 w148 w159 w172 w187 w204 w219 w231 w240 w247 w253 w263 w273 w283 w293 w303 w310 w318 w340 w351 w357 w365 w376 w391 w401 w411 w422 w439 w454] -> w34
              tunnel: w33 -> [w46 w61 w66 w71 w76 w86 w100 w121 w142 w148 w159 w172 w187 w204 w219 w231 w240 w247 w253 w263 w273 w283 w293 w303 w310 w318 w340 w351 w357 w365 w376 w391 w401 w411 w421 w438 w461]
              tunnel: [w41 w60 w65 w70 w81 w91 w105 w128 w145 w155 w165 w177 w192 w207 w217 w232 w237 w245 w252 w261 w271 w281 w291 w301 w309 w314 w337 w349 w356 w367 w378 w386 w396 w407 w427 w440 w463] -> w32
              event Timeout {
                n9 = event-data() -> ()  [unwired: 1 in, 1 out]
                n10 = while {
                  shift-right: [w57] -> _
                  shift-left: _ -> [w56]
                  tunnel: [w55] -> w44
                  stop <- TRUE stop-if-true
                  n11 = call <vilib>:"High Resolution Relative Seconds.vi"() -> ("relative seconds"=w57:dbl)
                  n12 = Subtract(x=w57, y=w56) -> (x-y=w55:dbl)
                }
                n13 = Unbundle By Name(w41) -> ("DAQ Status"=w40:T1)
                n14 = First Call?() -> (First Call?: T/F=w43:bool)
                n15 = Select(t=0.0, s=w43, f=w44) -> (s? t:f=→"Total (s)" →"Total Chart":dbl)
                n16 = case shown="\"created\", \"started\"" w40 {
                  tunnel: [w50 "" ("State(s) in Front (\"\")")] -> w39
                  frame "created", "started" {
                    n17 = call <userlib>:"Periodic Trigger__ogtk.vi"("time (ms)"=u32 1000) -> ("Triggered"=w52:bool)  [unwired: 12 in, 2 out]
                    n18 = Select(t="idle" ("State(s) in Front (\"\")"), s=w52, f="") -> (s? t:f=w50:string)
                  }
                  frame "idle", "stopped", "sweeping" {
                  }
                }
                n19 = call <vilib>:"Add State(s) to Queue__jki_lib_state_machine.vi"("State(s) in Front (\"\")"=w39, "State(s) in (\"\")"=w42) -> ("States Out"=w47:string)  [unwired: 13 in]
              }
              event Panel Close? {
                # "Discard the event because we'll close the front panel ourselves in Macro: Exit"
                # "Close Panel button (pressed) Event\n(this executes Macro: Exit to terminate the VI)"
                n20 = event-data() -> ()  [unwired: 1 in, 1 out]
                n21 = event-data("Discard?"=FALSE) -> ()  [unwired: 1 in, 1 out]
                n22 = call <vilib>:"Add State(s) to Queue__jki_lib_state_machine.vi"("State(s) in Front (\"\")"="//Macro: Exit", "State(s) in (\"\")"=w63) -> ("States Out"=w62:string)  [unwired: 13 in]
              }
              event User Event {
                n23 = event-data() -> ()  [unwired: 1 in, 5 out]
                n24 = call <vilib>:"Add State(s) to Queue__jki_lib_state_machine.vi"("State(s) in Front (\"\")"="Macro: Exit", "State(s) in (\"\")"=w68) -> ("States Out"=w67:string)  [unwired: 13 in]
              }
              event User Event {
                # "On Abort, no nice macro exit, but exit right away"
                n25 = event-data() -> ()  [unwired: 1 in, 5 out]
                n26 = call <vilib>:"Add State(s) to Queue__jki_lib_state_machine.vi"("State(s) in Front (\"\")"="Exit", "State(s) in (\"\")"=w73) -> ("States Out"=w72:string)  [unwired: 13 in]
              }
              event "DAQ AO": Value Change {
                n27 = event-data() -> ("NewVal"=w74:T5)  [unwired: 1 in]
                n28 = Unbundle By Name(w79) -> ("SMO"=w78:refnum<class "Instrument.DAQ.lvclass">)
                n29 = Bundle By Name(cluster=w78, "AO"=w74) -> (w77:refnum<class "Instrument.DAQ.lvclass">)
                n30 = local write "Method"("setAOconfig" ("String")) -> ()
                n31 = Bundle By Name(cluster=w79, "SMO"=w77) -> (w81:T19)
                n32 = call <vilib>:"Add State(s) to Queue__jki_lib_state_machine.vi"("State(s) in Front (\"\")"="Data: Process DAQ\nData: Process AO Channels" ("State(s) in Front (\"\")"), "State(s) in (\"\")"=w83) -> ("States Out"=w82:string)  [unwired: 13 in]
              }
              event "DAQ AI": Value Change {
                n33 = event-data() -> ("NewVal"=w84:T8)  [unwired: 1 in]
                n34 = local write "Method"("setAIconfig" ("String")) -> ()
                n35 = Unbundle By Name(w89) -> ("SMO"=w87:refnum<class "Instrument.DAQ.lvclass">)
                n36 = Bundle By Name(cluster=w87, "AI"=w84) -> (w88:refnum<class "Instrument.DAQ.lvclass">)
                n37 = Bundle By Name(cluster=w89, "SMO"=w88) -> (w91:T19)
                n38 = call <vilib>:"Add State(s) to Queue__jki_lib_state_machine.vi"("State(s) in Front (\"\")"="Data: Process DAQ\nData: Process AI Channels" ("State(s) in Front (\"\")"), "State(s) in (\"\")"=w93) -> ("States Out"=w92:string)  [unwired: 13 in]
              }
              event User Event {
                n39 = event-data() -> ("AO Configuration"=w99:T20)  [unwired: 1 in]
                "Payload" <- w99
                n40 = for {
                  tunnel: w99 -> [w108] mode=indexing
                  tunnel: [w109] -> w98 mode=concatenating
                  n41 = Unbundle By Name(w108) -> ("Channels"=w111:tag)
                  n42 = call <vilib>:"DAQmx Unflatten Channel String.vi"("names in"=w111) -> ("names out"=w110:string[])  [unwired: 13 in, 1 out]
                  n43 = for {
                    tunnel: w108 -> [w114]
                    tunnel: w110 -> [w113] mode=indexing
                    tunnel: [w112] -> w109 mode=indexing
                    n44 = Bundle By Name(cluster=w114, "Channels"=w113) -> (w112:T22)
                  }
                }
                n45 = local write "Method"("setAOconfig" ("String")) -> ()
                n46 = Unbundle By Name(w103) -> ("SMO"=w102:refnum<class "Instrument.DAQ.lvclass">)
                n47 = Bundle By Name(cluster=w102, "AO"=w99) -> (w101:refnum<class "Instrument.DAQ.lvclass">)
                n48 = First Call?() -> (First Call?: T/F=w97:bool)
                n49 = Bundle By Name(cluster=w103, "SMO"=w101) -> (w105:T19)
                n50 = local write "DAQ AO"(w98) -> ()
                n51 = Select(t="Data: Process DAQ" ("State(s) in Front (\"\")"), s=w97, f="Data: Process DAQ\nData: Process AO Channels" ("State(s) in Front (\"\")")) -> (s? t:f=w94:string)
                n52 = call <vilib>:"Add State(s) to Queue__jki_lib_state_machine.vi"("State(s) in Front (\"\")"=w94, "State(s) in (\"\")"=w107) -> ("States Out"=w106:string)  [unwired: 13 in]
              }
              event User Event {
                n53 = event-data() -> ("AI Configuration"=w120:T23, "Simulation mode"=w124:T24)  [unwired: 1 in]
                n54 = Bundle("AI Configuration"=w120, "Simulation mode"=w124) -> (w123:T25)  [unwired: 1 in]
                n55 = for {
                  tunnel: w120 -> [w133] mode=indexing
                  tunnel: [w131] -> w119 mode=concatenating
                  n56 = Unbundle By Name(w133) -> ("Channels"=w134:tag)
                  n57 = call <vilib>:"DAQmx Unflatten Channel String.vi"("names in"=w134) -> ("names out"=w132:string[])  [unwired: 13 in, 1 out]
                  n58 = for {
                    tunnel: w133 -> [w137]
                    tunnel: w132 -> [w136] mode=indexing
                    tunnel: [w135] -> w131 mode=indexing
                    n59 = Bundle By Name(cluster=w137, "Channels"=w136) -> (w135:T26)
                  }
                }
                n60 = Unbundle By Name(w126) -> ("SMO"=w122:refnum<class "Instrument.DAQ.lvclass">)
                n61 = local write "Payload"(w123) -> ()
                n62 = Bundle By Name(cluster=w122, "AI"=w120, "Simulation mode"=w124) -> (w125:refnum<class "Instrument.DAQ.lvclass">)
                n63 = local write "Method"("setAIconfig" ("String")) -> ()
                n64 = First Call?() -> (First Call?: T/F=w118:bool)
                n65 = Bundle By Name(cluster=w126, "SMO"=w125) -> (w128:T19)
                n66 = local write "DAQ AI"(w119) -> ()
                n67 = Select(t="Data: Process DAQ" ("State(s) in Front (\"\")"), s=w118, f="Data: Process DAQ\nData: Process AI Channels" ("State(s) in Front (\"\")")) -> (s? t:f=w116:string)
                n68 = call <vilib>:"Add State(s) to Queue__jki_lib_state_machine.vi"("State(s) in Front (\"\")"=w116, "State(s) in (\"\")"=w130) -> ("States Out"=w129:string)  [unwired: 13 in]
              }
              event User Event {
                n69 = event-data() -> ("AO Channels"=w139:T27)  [unwired: 1 in]
                n70 = local write "Method"("setAO" ("String")) -> ()
                n71 = local write "Payload"(w139) -> ()
                n72 = Unbundle By Name(w143) -> ("SMO"=w141:refnum<class "Instrument.DAQ.lvclass">)
                n73 = Bundle By Name(cluster=w141, "Cfg_AO"=w139) -> (w138:refnum<class "Instrument.DAQ.lvclass">)
                n74 = Bundle By Name(cluster=w143, "SMO"=w138) -> (w145:T19)
                n75 = call <vilib>:"Add State(s) to Queue__jki_lib_state_machine.vi"("State(s) in Front (\"\")"="Data: Process AO Channels" ("State(s) in Front (\"\")"), "State(s) in (\"\")"=w147) -> ("States Out"=w146:string)  [unwired: 13 in]
              }
              event User Event {
                n76 = event-data() -> ("AI Channels"=w151:T30)  [unwired: 1 in]
                n77 = Unbundle By Name(w153) -> ("SMO"=w152:refnum<class "Instrument.DAQ.lvclass">)
                n78 = Bundle By Name(cluster=w152, "Cfg_AI"=w151) -> (w149:refnum<class "Instrument.DAQ.lvclass">)
                n79 = local write "Payload"(w151) -> ()
                n80 = local write "Method"("setAI" ("String")) -> ()
                n81 = Bundle By Name(cluster=w153, "SMO"=w149) -> (w155:T19)
                n82 = call <vilib>:"Add State(s) to Queue__jki_lib_state_machine.vi"("State(s) in Front (\"\")"="Data: Process AI Channels" ("State(s) in Front (\"\")"), "State(s) in (\"\")"=w157) -> ("States Out"=w156:string)  [unwired: 13 in]
              }
              event User Event {
                n83 = event-data() -> ("REF Channels"=w161:T32)  [unwired: 1 in]
                n84 = local write "Method"("setREF" ("String")) -> ()
                n85 = local write "Payload"(w161) -> ()
                n86 = Unbundle By Name(w163) -> ("SMO"=w162:refnum<class "Instrument.DAQ.lvclass">)
                n87 = Bundle By Name(cluster=w162, "Cfg_REF"=w161) -> (w160:refnum<class "Instrument.DAQ.lvclass">)
                n88 = Bundle By Name(cluster=w163, "SMO"=w160) -> (w165:T19)
                n89 = call <vilib>:"Add State(s) to Queue__jki_lib_state_machine.vi"("State(s) in Front (\"\")"="Data: Process REF Channels" ("State(s) in Front (\"\")"), "State(s) in (\"\")"=w167) -> ("States Out"=w166:string)  [unwired: 13 in]
              }
              event User Event {
                n90 = event-data() -> ("Input Gain"=w169:dbl[])  [unwired: 1 in]
                n91 = for {
                  tunnel: T9 {"Channel"="", "Gain"=0.0} ("System Cluster") -> [w182]
                  tunnel: w169 -> [w181] mode=indexing
                  tunnel: [w180] -> w168 mode=indexing
                  n92 = Bundle By Name(cluster=w182, "Gain"=w181) -> (w180:T9)
                }
                n93 = local write "Method"("setInputGain" ("String")) -> ()
                n94 = Unbundle By Name(w175) -> ("SMO"=w174:refnum<class "Instrument.DAQ.lvclass">)
                n95 = Bundle By Name(cluster=w174, "Gain_AI"=w168) -> (w173:refnum<class "Instrument.DAQ.lvclass">)
                n96 = local write "Payload"(w169) -> ()
                n97 = Bundle By Name(cluster=w175, "SMO"=w173) -> (w177:T19)
                n98 = call <vilib>:"Add State(s) to Queue__jki_lib_state_machine.vi"("State(s) in Front (\"\")"="Data: Process Input Gain" ("State(s) in Front (\"\")"), "State(s) in (\"\")"=w179) -> ("States Out"=w178:string)  [unwired: 13 in]
              }
              event User Event {
                n99 = event-data() -> ("Input Offset"=w184:dbl[])  [unwired: 1 in]
                n100 = for {
                  tunnel: T9 {"Channel"="", "Gain"=0.0} ("System Cluster") -> [w197]
                  tunnel: w184 -> [w196] mode=indexing
                  tunnel: [w195] -> w183 mode=indexing
                  n101 = Bundle By Name(cluster=w197, "Gain"=w196) -> (w195:T9)
                }
                n102 = local write "Method"("setInputOffset" ("String")) -> ()
                n103 = Unbundle By Name(w190) -> ("SMO"=w189:refnum<class "Instrument.DAQ.lvclass">)
                n104 = Bundle By Name(cluster=w189, "Offset_AI"=w183) -> (w188:refnum<class "Instrument.DAQ.lvclass">)
                n105 = local write "Payload"(w184) -> ()
                n106 = Bundle By Name(cluster=w190, "SMO"=w188) -> (w192:T19)
                n107 = call <vilib>:"Add State(s) to Queue__jki_lib_state_machine.vi"("State(s) in Front (\"\")"="Data: Process Input Offset" ("State(s) in Front (\"\")"), "State(s) in (\"\")"=w194) -> ("States Out"=w193:string)  [unwired: 13 in]
              }
              event User Event {
                n108 = event-data() -> ("Input Gain"=w199:dbl[])  [unwired: 1 in]
                n109 = for {
                  tunnel: T9 {"Channel"="", "Gain"=0.0} ("System Cluster") -> [w212]
                  tunnel: w199 -> [w211] mode=indexing
                  tunnel: [w210] -> w198 mode=indexing
                  n110 = Bundle By Name(cluster=w212, "Gain"=w211) -> (w210:T9)
                }
                n111 = local write "Method"("setOutputGain" ("String")) -> ()
                n112 = local write "Payload"(w199) -> ()
                n113 = Unbundle By Name(w205) -> ("SMO"=w203:refnum<class "Instrument.DAQ.lvclass">)
                n114 = Bundle By Name(cluster=w203, "Gain_AO"=w198) -> (w202:refnum<class "Instrument.DAQ.lvclass">)
                n115 = Bundle By Name(cluster=w205, "SMO"=w202) -> (w207:T19)
                n116 = call <vilib>:"Add State(s) to Queue__jki_lib_state_machine.vi"("State(s) in Front (\"\")"="Data: Process Output Gain" ("State(s) in Front (\"\")"), "State(s) in (\"\")"=w209) -> ("States Out"=w208:string)  [unwired: 13 in]
              }
              event User Event {
                w215 = 10123 items=["Finite Samples"=10178, "Continuous Samples"=10123, "Hardware Timed Single Point"=12522] ("sample mode")
                n117 = event-data() -> ("Sampling"=w214:T34)  [unwired: 1 in]
                n118 = local write "Payload"(w214) -> ()
                n119 = local write "Method"("setSampling" ("String")) -> ()
                n120 = Unbundle By Name(w221) -> ("SMO"=w220:refnum<class "Instrument.DAQ.lvclass">)
                n121 = Bundle By Name(cluster=w214, "sample mode"=w215) -> (w213:T34)
                n122 = Bundle By Name(cluster=w220, "Sampling"=w213) -> (w218:refnum<class "Instrument.DAQ.lvclass">)
                n123 = Bundle By Name(cluster=w221, "SMO"=w218) -> (w217:T19)
                n124 = call <vilib>:"Add State(s) to Queue__jki_lib_state_machine.vi"("State(s) in Front (\"\")"="Data: Process Sampling" ("State(s) in Front (\"\")"), "State(s) in (\"\")"=w224) -> ("States Out"=w223:string)  [unwired: 13 in]
              }
              event User Event {
                n125 = event-data() -> ("setSweep"=w226:T37)  [unwired: 1 in]
                n126 = local write "Method"("setSweep" ("String")) -> ()
                n127 = local write "Payload"(w226) -> ()
                n128 = Unbundle By Name(w230) -> ("SMO"=w229:refnum<class "Instrument.DAQ.lvclass">)
                n129 = Bundle By Name(cluster=w229, "Sweep"=w226) -> (w228:refnum<class "Instrument.DAQ.lvclass">)
                n130 = Bundle By Name(cluster=w230, "SMO"=w228) -> (w232:T19)
                n131 = call <vilib>:"Add State(s) to Queue__jki_lib_state_machine.vi"("State(s) in Front (\"\")"="Data: Process Sweep" ("State(s) in Front (\"\")"), "State(s) in (\"\")"=w234) -> ("States Out"=w233:string)  [unwired: 13 in]
              }
              event User Event {
                n132 = event-data() -> ("measureOffset"=w236:T41)  [unwired: 1 in]
                n133 = local write "Method"("measureOffset" ("String")) -> ()
                n134 = Bundle By Name(cluster=w238, "Measure Offset"=w236) -> (w237:T19)
                n135 = local write "Measure Offset"(w236) -> ()
                n136 = call <vilib>:"Add State(s) to Queue__jki_lib_state_machine.vi"("State(s) in Front (\"\")"="DSP: Zero DAQ Offset\nData: Zero Amplitude\nDSP: Measure DAQ Offset\nData: Restore Amplitude" ("State(s) in Front (\"\")"), "State(s) in (\"\")"=w242) -> ("States Out"=w241:string)  [unwired: 13 in]
              }
              event User Event {
                n137 = event-data() -> ("Reset Phase"=w244:T42)  [unwired: 1 in]
                n138 = local write "Method"("zeroPhase" ("String")) -> ()
                n139 = Bundle By Name(cluster=w246, "Measure Offset"=w244) -> (w245:T19)
                n140 = local write "Reset Phase"(w244) -> ()
                n141 = call <vilib>:"Add State(s) to Queue__jki_lib_state_machine.vi"("State(s) in (\"\")"=w249) -> ("States Out"=w248:string)  [unwired: 14 in]
              }
              event User Event {
                w251 = "DAQ: AUTO" ("State(s) in Front (\"\")")
                n142 = event-data() -> ()  [unwired: 1 in, 5 out]
                n143 = local write "Method"("autoConfigureDAQ" ("String")) -> ()
                n144 = local write "Payload"(w251) -> ()
                n145 = call <vilib>:"Add State(s) to Queue__jki_lib_state_machine.vi"("State(s) in Front (\"\")"=w251, "State(s) in (\"\")"=w255) -> ("States Out"=w254:string)  [unwired: 13 in]
              }
              event User Event {
                # "#todo\n????"
                n146 = event-data() -> ("PreFilter"=w257:T43)  [unwired: 1 in, 4 out]
                n147 = local write "Payload"(w257) -> ()
                n148 = Unbundle By Name(w260) -> ("SMO"=w259:refnum<class "Instrument.DAQ.lvclass">)
                n149 = Bundle By Name(cluster=w259, "Prefilter"=w257) -> (w258:refnum<class "Instrument.DAQ.lvclass">)
                n150 = local write "Method"("setPreFilter" ("String")) -> ()
                n151 = Bundle By Name(cluster=w260, "SMO"=w258) -> (w261:T19)
                n152 = call <vilib>:"Add State(s) to Queue__jki_lib_state_machine.vi"("State(s) in Front (\"\")"="" ("State(s) in Front (\"\")"), "State(s) in (\"\")"=w265) -> ("States Out"=w264:string)  [unwired: 13 in]
              }
              event User Event {
                n153 = event-data() -> ("Amplitude Limit"=w267:T44)  [unwired: 1 in, 4 out]
                n154 = Unbundle By Name(w270) -> ("SMO"=w269:refnum<class "Instrument.DAQ.lvclass">)
                n155 = Bundle By Name(cluster=w269, "Amplitude Limit"=w267) -> (w268:refnum<class "Instrument.DAQ.lvclass">)
                n156 = local write "Method"("setAmplitudeLimit" ("String")) -> ()
                n157 = local write "Payload"(w267) -> ()
                n158 = Bundle By Name(cluster=w270, "SMO"=w268) -> (w271:T19)
                n159 = call <vilib>:"Add State(s) to Queue__jki_lib_state_machine.vi"("State(s) in Front (\"\")"="Data: Process AO Channels" ("State(s) in Front (\"\")"), "State(s) in (\"\")"=w275) -> ("States Out"=w274:string)  [unwired: 13 in]
              }
              event User Event {
                n160 = event-data() -> ("DC Limit"=w277:T45)  [unwired: 1 in, 4 out]
                n161 = Unbundle By Name(w280) -> ("SMO"=w279:refnum<class "Instrument.DAQ.lvclass">)
                n162 = Bundle By Name(cluster=w279, "DC Limit"=w277) -> (w278:refnum<class "Instrument.DAQ.lvclass">)
                n163 = local write "Method"("setDCLimit" ("String")) -> ()
                n164 = local write "Payload"(w277) -> ()
                n165 = Bundle By Name(cluster=w280, "SMO"=w278) -> (w281:T19)
                n166 = call <vilib>:"Add State(s) to Queue__jki_lib_state_machine.vi"("State(s) in Front (\"\")"="Data: Process AO Channels" ("State(s) in Front (\"\")"), "State(s) in (\"\")"=w285) -> ("States Out"=w284:string)  [unwired: 13 in]
              }
              event User Event {
                n167 = event-data() -> ("Duty Cycle"=w287:T46)  [unwired: 1 in, 4 out]
                n168 = Unbundle By Name(w290) -> ("SMO"=w289:refnum<class "Instrument.DAQ.lvclass">)
                n169 = Bundle By Name(cluster=w289, "Duty Cycle"=w287) -> (w288:refnum<class "Instrument.DAQ.lvclass">)
                n170 = local write "Method"("setDutyCycle" ("String")) -> ()
                n171 = local write "Payload"(w287) -> ()
                n172 = Bundle By Name(cluster=w290, "SMO"=w288) -> (w291:T19)
                n173 = call <vilib>:"Add State(s) to Queue__jki_lib_state_machine.vi"("State(s) in Front (\"\")"="Data: Process AO Channels" ("State(s) in Front (\"\")"), "State(s) in (\"\")"=w295) -> ("States Out"=w294:string)  [unwired: 13 in]
              }
              event User Event {
                n174 = event-data() -> ("Link Frequencies"=w297:T47)  [unwired: 1 in, 4 out]
                n175 = Unbundle By Name(w300) -> ("SMO"=w299:refnum<class "Instrument.DAQ.lvclass">)
                n176 = Bundle By Name(cluster=w299, "Link Frequencies"=w297) -> (w298:refnum<class "Instrument.DAQ.lvclass">)
                n177 = local write "Method"("setLinkFrequencies" ("String")) -> ()
                n178 = local write "Payload"(w297) -> ()
                n179 = Bundle By Name(cluster=w300, "SMO"=w298) -> (w301:T19)
                n180 = call <vilib>:"Add State(s) to Queue__jki_lib_state_machine.vi"("State(s) in Front (\"\")"="Data: Process AO Channels\nData: Process REF Channels" ("State(s) in Front (\"\")"), "State(s) in (\"\")"=w305) -> ("States Out"=w304:string)  [unwired: 13 in]
              }
              event User Event {
                n181 = event-data() -> ()  [unwired: 1 in, 5 out]
                n182 = local write "Method"("zeroOffset" ("String")) -> ()
                n183 = local write "Zero Offset"(TRUE ("zero offset")) -> ()
                n184 = call <vilib>:"Add State(s) to Queue__jki_lib_state_machine.vi"("State(s) in Front (\"\")"="DSP: Zero DAQ Offset" ("State(s) in Front (\"\")"), "State(s) in (\"\")"=w312) -> ("States Out"=w311:string)  [unwired: 13 in]
              }
              event User Event {
                # "start: Start acquisition (Macro: Acquire)\nstop: Stop acquisition (Macro: Stop)\nreset: Stop and Start acquisition (Macro: Stop, Macro: Start)\n\nif already running:\n- the private events setAOconfig, setAIconfig, setSampling\nwill be written to data cluster, but otherwise will be ignored until\nacquisition is reset\n- setAO and setREF will be implemented on next Acquisition iteration"
                n185 = event-data() -> ("setState"=w315:T48)  [unwired: 1 in]
                n186 = Unbundle By Name(w314) -> ("DAQ Status"=w316:T1)
                n187 = local write "Payload"(w315) -> ()
                n188 = local write "Method"("setState" ("String")) -> ()
                n189 = case shown="\"stop sweep\"" w315 {
                  tunnel: w316 -> [w322 _ w331 _ _]
                  tunnel: [w321 "Generator: Stop\nMacro: Stop DAQmx" ("State(s) in Front (\"\")") w327 w332 "Generator: Stop Sweep" ("format string")] -> w313
                  frame "start", Default {
                    n190 = case shown="Default" w322 {
                      tunnel: ["" ("State(s) in Front (\"\")") "Generator: Start\nMacro: Start DAQmx" ("State(s) in Front (\"\")")] -> w321
                      frame "created", "started" {
                      }
                      frame Default {
                      }
                    }
                  }
                  frame "stop" {
                  }
                  frame "reset" {
                    n191 = Equal?(x=Status--enum."idle" ("state"), y=w331) -> (x = y?=w330:bool)
                    n192 = Select(t="Data: Clear Sweep Data", s=w330, f="Macro: Stop DAQmx\nGenerator: Stop\nGenerator: Start\nMacro: Start DAQmx" ("State(s) in Front (\"\")")) -> (s? t:f=w327:string)
                    "reset" <- w327
                  }
                  frame "start sweep" {
                    w332 = "Sweep: Initialize\nData: Clear Sweep Data\nGenerator: Start Sweep" ("format string")
                    "start sweep" <- w332
                  }
                  frame "stop sweep" {
                  }
                }
                n193 = call <vilib>:"Add State(s) to Queue__jki_lib_state_machine.vi"("State(s) in (\"\")"=w320, "State(s) at Back (\"\")"=w313) -> ("States Out"=w319:string)  [unwired: 13 in]
              }
              event User Event {
                n194 = event-data() -> ("setCalibration"=w334:T14)  [unwired: 1 in, 4 out]
                n195 = local write "Method"("setCalibration" ("String")) -> ()
                n196 = local write "Payload"(w334) -> ()
                n197 = Format Into String(w334) -> (resulting string=w335:string)  [unwired: 3 in, 1 out]
                n198 = call <vilib>:"Build State String with Arguments__JKI_lib_State_Machine.vi"("Arguments (\"\")"=w335, "State"="DAQ: CALIBRATE" ("State(s) in Front (\"\")")) -> ("State with Arguments"=w338:string)  [unwired: 4 in]
                n199 = call <vilib>:"Add State(s) to Queue__jki_lib_state_machine.vi"("State(s) in (\"\")"=w342, "State(s) at Back (\"\")"=w338) -> ("States Out"=w341:string)  [unwired: 13 in]
              }
              event User Event {
                n200 = event-data() -> ("showDAQUI"=w347:T49)  [unwired: 1 in, 4 out]
                n201 = local write "Method"("showUI" ("String")) -> ()
                n202 = Select(t="Open", s=w347, f="Close") -> (s? t:f=w344:string)
                n203 = local write "Payload"(w344) -> ()
                n204 = call <vilib>:"Build State String with Arguments__JKI_lib_State_Machine.vi"("Arguments (\"\")"=w344, "State"="UI: Front Panel State" ("State(s) in Front (\"\")")) -> ("State with Arguments"=w343:string)  [unwired: 4 in]
                n205 = call <vilib>:"Add State(s) to Queue__jki_lib_state_machine.vi"("State(s) in Front (\"\")"=w343, "State(s) in (\"\")"=w353) -> ("States Out"=w352:string)  [unwired: 13 in]
              }
              event User Event {
                n206 = event-data() -> ("Status"=w354:T2)  [unwired: 1 in, 4 out]
                "DAQmx Status" <- w354
                n207 = local write "Method"("DAQmx.Status" ("String")) -> ()
                n208 = Bundle By Name(cluster=w358, "DAQmx Status"=w354) -> (w356:T19)
                n209 = call <vilib>:"Add State(s) to Queue__jki_lib_state_machine.vi"("State(s) in Front (\"\")"="Data: Process State >> -DAQmx" ("State(s) in Front (\"\")"), "State(s) in (\"\")"=w360) -> ("States Out"=w361:string)  [unwired: 13 in]
              }
              event User Event {
                n210 = event-data() -> ("Devices"=w362:T50[])  [unwired: 1 in, 4 out]
                n211 = local write "Payload"(w362) -> ()
                n212 = local write "Method"("DAQmx.Devices" ("String")) -> ()
                n213 = Unbundle By Name(w366) -> ("SMO"=w368:refnum<class "Instrument.DAQ.lvclass">)
                n214 = Bundle By Name(cluster=w368, "Devices"=w362) -> (w364:refnum<class "Instrument.DAQ.lvclass">)
                n215 = Bundle By Name(cluster=w366, "SMO"=w364) -> (w367:T19)
                n216 = call <vilib>:"Add State(s) to Queue__jki_lib_state_machine.vi"("State(s) in Front (\"\")"="Data: Process Devices >> -DAQmx" ("State(s) in Front (\"\")"), "State(s) in (\"\")"=w370) -> ("States Out"=w371:string)  [unwired: 13 in]
              }
              event User Event {
                n217 = event-data() -> ("Calibration out"=w372:T51)  [unwired: 1 in, 4 out]
                n218 = call "Convert DAQmx to DAQ cal.vi"("Calibration in"=w372) -> ("Array"=w373:T52[])  [unwired: 10 in]
                n219 = local write "Payload"(w372) -> ()
                n220 = local write "Method"("DAQmx.Calibration" ("String")) -> ()
                n221 = Unbundle By Name(w377) -> ("SMO"=w379:refnum<class "Instrument.DAQ.lvclass">)
                n222 = Bundle By Name(cluster=w379, "Calibration"=w373) -> (w374:refnum<class "Instrument.DAQ.lvclass">)
                n223 = Bundle By Name(cluster=w377, "SMO"=w374) -> (w378:T19)
                n224 = call <vilib>:"Add State(s) to Queue__jki_lib_state_machine.vi"("State(s) in Front (\"\")"="Data: Process Calibration >> -DAQmx" ("State(s) in Front (\"\")"), "State(s) in (\"\")"=w381) -> ("States Out"=w382:string)  [unwired: 13 in]
              }
              event User Event {
                n225 = event-data() -> ("Fs"=w384:dbl, "#s"=w383:i32)  [unwired: 1 in]
                n226 = local write "Method"("DAQmx.Timing" ("String")) -> ()
                n227 = Unbundle By Name(w387) -> ("SMO"=w389:refnum<class "Instrument.DAQ.lvclass">)
                n228 = Bundle By Name(cluster=w389, "Fs"=w384, "#s"=w383) -> (w388:refnum<class "Instrument.DAQ.lvclass">)
                n229 = local write "Payload"(w384) -> ()
                n230 = Bundle By Name(cluster=w387, "SMO"=w388) -> (w386:T19)
                n231 = call <vilib>:"Add State(s) to Queue__jki_lib_state_machine.vi"("State(s) in Front (\"\")"="Data: Process Sampling >> -DAQmx" ("State(s) in Front (\"\")"), "State(s) in (\"\")"=w392) -> ("States Out"=w393:string)  [unwired: 13 in]
              }
              event User Event {
                n232 = event-data() -> ("AOconfig"=w394:T53)  [unwired: 1 in, 4 out]
                n233 = Unbundle By Name(w395) -> ("SMO"=w398:refnum<class "Instrument.DAQ.lvclass">)
                n234 = Bundle By Name(cluster=w398, "AO"=w394) -> (w397:refnum<class "Instrument.DAQ.lvclass">)
                n235 = local write "Method"("DAQmx.AOconfig" ("String")) -> ()
                n236 = local write "Payload"(w394) -> ()
                n237 = Bundle By Name(cluster=w395, "SMO"=w397) -> (w396:T19)
                n238 = call <vilib>:"Add State(s) to Queue__jki_lib_state_machine.vi"("State(s) in Front (\"\")"="Data: Process DAQ >> -DAQmx\nData: Process AO Channels >> -DAQmx" ("State(s) in Front (\"\")"), "State(s) in (\"\")"=w402) -> ("States Out"=w403:string)  [unwired: 13 in]
              }
              event User Event {
                n239 = event-data() -> ("AIconfig"=w404:T57)  [unwired: 1 in, 4 out]
                n240 = local write "Payload"(w404) -> ()
                n241 = Unbundle By Name(w406) -> ("SMO"=w409:refnum<class "Instrument.DAQ.lvclass">)
                n242 = Bundle By Name(cluster=w409, "AI"=w404) -> (w408:refnum<class "Instrument.DAQ.lvclass">)
                n243 = local write "Method"("DAQmx.AIconfig" ("String")) -> ()
                n244 = Bundle By Name(cluster=w406, "SMO"=w408) -> (w407:T19)
                n245 = call <vilib>:"Add State(s) to Queue__jki_lib_state_machine.vi"("State(s) in Front (\"\")"="Data: Process DAQ >> -DAQmx\nData: Process AI Channels >> -DAQmx" ("State(s) in Front (\"\")"), "State(s) in (\"\")"=w412) -> ("States Out"=w413:string)  [unwired: 13 in]
              }
              event User Event {
                n246 = event-data() -> ("AO"=w417:waveform(dbl)[], "AI"=w414:waveform(dbl)[], "REF_X"=w416:waveform(dbl)[], "REF_Y"=w415:waveform(dbl)[])  [unwired: 1 in, 4 out]
                n247 = Unbundle By Name(w426) -> ("SMO"=w423:refnum<class "Instrument.DAQ.lvclass">)
                n248 = local write "Method"("DAQmx.Waveforms" ("String")) -> ()
                n249 = call "Multiply Waveform by Output Gain.vi"("WFM in"=w417, "Instrument.DAQ"=w423) -> ("error out"=w419:errorcluster, "WFM out"=w424:waveform(dbl)[])  [unwired: 7 in, 1 out]
                n250 = call "Divide Waveform by Input Gain.vi"("WFM in"=w414, "Instrument.DAQ"=w423) -> ("error out"=w420:errorcluster, "WFM out"=w418:waveform(dbl)[])  [unwired: 7 in, 1 out]
                n251 = Bundle By Name(cluster=w423, "AO"=w424, "AI"=w418, "REF_X"=w416, "REF_Y"=w415) -> (w428:refnum<class "Instrument.DAQ.lvclass">)
                n252 = Merge Errors(w421, w420, w419) -> (w422:errorcluster)
                n253 = Bundle By Name(cluster=w426, "SMO"=w428) -> (w427:T19)
                n254 = call <vilib>:"Add State(s) to Queue__jki_lib_state_machine.vi"("State(s) in Front (\"\")"="Macro: DSP" ("State(s) in Front (\"\")"), "State(s) in (\"\")"=w430) -> ("States Out"=w431:string)  [unwired: 13 in]
              }
              event User Event {
                # "report sweeping when a sweep starts."
                n255 = event-data() -> ("sweep status"=w441:T13)  [unwired: 1 in]
                n256 = Format Into String(w441) -> (resulting string=→"sweep status":string)  [unwired: 3 in, 1 out]
                n257 = case shown="\"sweeping\"" w441 {
                  tunnel: [Status--enum."started" ("status") Status--enum."sweeping" ("status")] -> w435
                  frame Default {
                  }
                  frame "sweeping" {
                  }
                }
                n258 = local write "Method"("Generator.SweepState" ("String")) -> ()
                n259 = Unbundle By Name(w440) -> ("SMO"=w442:refnum<class "Instrument.DAQ.lvclass">)
                n260 = call "Is Value Changed.vim"("value"=w435) -> ("changed or first call?"=w433:bool)
                n261 = Equal?(x=w435, y=Status--enum."sweeping" ("status")) -> (x = y?=w434:bool)
                n262 = And(x=w433, y=w434) -> (x .and. y?=w432:bool)
                n263 = case shown="True" w432 {
                  tunnel: w442 -> [_ w451]
                  tunnel: w435 -> [_ w450]
                  tunnel: [w447 w449] -> w439
                  tunnel: w438 -> [w447 w448]
                  frame False {
                  }
                  frame True {
                    n264 = call "DAQ.getDAQState.vi"("error in (no error)"=w448, "status"=w450, "Instrument.DAQ"=w451) -> ("error out"=w449:errorcluster)  [unwired: 7 in, 1 out]
                  }
                }
                n265 = call <userlib>:"MGI Milliseconds Since Last Call.vi"() -> ("ms"=→"Generate (ms)" →"Generator Chart":u32)  [unwired: 6 in, 1 out]
                n266 = call <vilib>:"Add State(s) to Queue__jki_lib_state_machine.vi"("State(s) in (\"\")"=w445) -> ("States Out"=w444:string)  [unwired: 14 in]
              }
              event User Event {
                n267 = event-data() -> ("AO Channels"=w465:T61)  [unwired: 1 in, 4 out]
                n268 = Unbundle By Name(w462) -> ("SMO"=w464:refnum<class "Instrument.DAQ.lvclass">)
                n269 = local write "Method"("Generator.AOchannels" ("String")) -> ()
                n270 = call "Merge AO Settings from Generator.vi"("error in (no error)"=w461, "configuration.AO Channels"=w465, "Instrument.DAQ in"=w464) -> ("error out"=w455:errorcluster, "Instrument.DAQ out"=w457:refnum<class "Instrument.DAQ.lvclass">)  [unwired: 7 in]
                n271 = call "Multiply Amplitude and Offset by Output Gain.vi"("error in (no error)"=w455, "Instrument.DAQ"=w457) -> ("error out"=w454:errorcluster, "Instrument.DAQ out"=w456:refnum<class "Instrument.DAQ.lvclass">)  [unwired: 8 in]
                n272 = Bundle By Name(cluster=w462, "SMO"=w456) -> (w463:T19)
                n273 = call <vilib>:"Add State(s) to Queue__jki_lib_state_machine.vi"("State(s) in Front (\"\")"="Data: Update AO Channels" ("States Out"), "State(s) in (\"\")"=w459) -> ("States Out"=w460:string)  [unwired: 13 in]
              }
            }
          }
          frame "---------- Core ----------" {
            # "Do not put any code in this frame.\n(it is a separator no-op)"
            n274 = call <vilib>:"Add State(s) to Queue__jki_lib_state_machine.vi"("State(s) in (\"\")"=w471) -> ("States Out"=w470:string)  [unwired: 14 in]
          }
          frame Default {
            w482 = 42 items=["No error", "Argument error", "Memory is full", "Out of zone", "End of file", "File already open", "Generic file I/O error", "File not found", "File permission error", "Disk is full", "Duplicate path", "Too many files open", "System feature not enabled", "Resource file not found", "Cannot add resource", "Resource not found", "Image not found", "Image memory error", "Pen does not exist", "Config type invalid", "Config token not found", "Config parse error", "Config memory error", "Bad external code format", "Bad external code offset", "External code not present", "Null window", "Destroy window error", "Null menu", "Print aborted", "Bad print record", "Print driver error", "Windows error during printing", "Memory error during printing", "Print dialog error", "Generic print error", "Invalid device refnum", "Device not found", "Device parameter error", "Device unit error", "Cannot open device", "Device call aborted", "Generic error", "Cancelled by user", "Object ID too low", "Object ID too high", "Object not in heap", "Unknown heap", "Unknown object (invalid DefProc)", "Unknown object (DefProc not in table)", "Message out of range", "Invalid (null) method", "Unknown message", "Manager call not supported", "Bad address", "Network operation in progress", "Network operation timed out", "Connection is busy", "Network attribute not supported", "Network error", "Address in use", "System out of memory", "Connection aborted", "Connection refused", "Not connected", "Already connected", "Connection closed", "Initialization error (interapplication manager)", "Bad occurrence", "Wait on unbound occurrence handler", "Occurrence queue overflow", "Datalog type conflict", "Unused", "Unrecognized type (interapplication manager)", "Memory corrupt", "Failed to make temporary DLL", "Old CIN version", "Drag socket not found", "Failed to load drop-object", "Failed to register OLE object", "Failed to release OLE object", "Format specifier type mismatch", "Unknown format specifier", "Too few format specifiers", "Too many format specifiers", "Scan failed", "Newer CIN version", "Error converting to variant", "Runtime menu error", "Password tampered", "Variant attribute not found", "Incompatible variant data type", "Event data is not available", "Event Store is not present", "Occurrence is not found", "Event Queue is not created", "Event info is not available", "Refnum passed is NULL", "Error retrieving Class GUID", "Error retrieving CoClass GUID", "Error retrieving TypeLib GUID.", "Bad built application magic bytes.", "Specific driver is different from the specific driver associated with the Logical Name.", "There is no session opened to the class driver.", "Max Error", "MAX - Error with config objects", "MAX - Error loading configuration", "MAX - Group not supported"]
            # "Current State"
            # "Do not delete, rename, or modify this frame.\n(this is used to capture unhandled states and typos)"
            # "Handle mistyped state name (developer tool)"
            n275 = Format Into String(format string="Software Exception: Unhandled State \"%s\"." ("message"), error in=w478, w473) -> (resulting string=w481:string, error out=w480:errorcluster)  [unwired: 1 in]
            n276 = call <vilib>:"Error Cluster From Error Code.vi"("show call chain? (False)"=TRUE, "error in (no error)"=w480, "error message (\"\")"=w481, "error code (0)"=w482) -> ("error out"=w479:errorcluster)  [unwired: 5 in]
            n277 = call <vilib>:"Add State(s) to Queue__jki_lib_state_machine.vi"("State(s) in (\"\")"=w477) -> ("States Out"=w476:string)  [unwired: 14 in]
          }
          frame "Initialize Core Data" {
            # "Do not delete, rename, or modify this frame.\n(this is used to determine panel behavior on exit)"
            # "originally closed?"
            # "exe?"
            # "If panel starts closed or is an EXE, then close it when we exit"
            n278 = property class="VI"() -> ("Front Panel.Open"=w492:bool)  [unwired: 2 in, 2 out]
            n279 = property class="App"() -> ("App.Kind"=w491:T10)  [unwired: 2 in, 2 out]
            n280 = control-ref of="Current VI Reference"() -> (w485:refnum<vi>)
            n281 = Not(x=w492) -> (.not. x?=w489:bool)
            n282 = Equal?(x=w491, y=T10."Run Time System" ("Application:Kind")) -> (x = y?=w488:bool)
            n283 = Or(x=w489, y=w488) -> (x .or. y?=w486:bool)
            n284 = Bundle By Name(cluster=w487, "Core.Current VI Reference"=w485, "Core.Close Panel on Exit?"=w486) -> (w494:T19)
            n285 = call <vilib>:"Add State(s) to Queue__jki_lib_state_machine.vi"("State(s) in (\"\")"=w496) -> ("States Out"=w495:string)  [unwired: 14 in]
          }
          frame "Error Handler" {
            w503 = FALSE  # Stop on Unhandled Error (T)
            # "Clear error"
            # "There was an error while handling the error.\nStop the process. This error can only occur if public events references are invalid or if the state machine object is destroyed."
            n286 = Unbundle By Name(w507) -> ("SMO"=w500:refnum<class "Instrument.DAQ.lvclass">)
            n287 = call-dynamic "Handle Error.vi"("Stop on Unhandled Error (T)"=w503, "error in"=w499, "SMO"=w500) -> ("handling error"=w504:errorcluster, "Unhandled error"=w501:errorcluster)  [unwired: 6 in, 1 out]
            n288 = Bundle By Name(cluster=w507, "Core.Last Error.remaining states"=w498, "Core.Last Error.error"=w501) -> (w506:T19)
            n289 = Select(t="Exit", s=w504, f="Macro: Post Error Handling") -> (s? t:f=w502:string)
          }
          frame "Exit" {
            # "Do not put any code in this frame.\n(No errors that occur here will be handled.)"
            n290 = Unbundle By Name(w511) -> ("Core.Last Error.error"=w510:errorcluster)
            n291 = call <vilib>:"Add State(s) to Queue__jki_lib_state_machine.vi"("State(s) in (\"\")"=w515) -> ("States Out"=w514:string)  [unwired: 14 in]
          }
          frame "---------- Data ----------" {
            # "Do not put any code in this frame.\n(It is a separator no-op. You can make a copy of this frame to create a new Data frame)"
            n292 = call <vilib>:"Add State(s) to Queue__jki_lib_state_machine.vi"("State(s) in (\"\")"=w520) -> ("States Out"=w519:string)  [unwired: 14 in]
          }
          frame "Data: Initialize" {
            w521 = Generator.Sweep_Status--enum."stopping"  # Sweep Status
            w522 = dbl[] []  # Saved Amplitudes
            w523 = DAQmx.Status--enum."idle"  # DAQmx Status
            w526 = T64 {"Current VI Reference"=refnum, "Close Panel on Exit?"=FALSE, "Last Error"={"error"={"status"=FALSE, "code"=0, "source"=""}, "previous state"="", "remaining states"=""}, "Shutdown?"=FALSE}  # Core
            w525 = T11 {"AO"=[], "AI"=[], "X"=[], "Y"=[]}  # SweepWaveforms
            w529 = FALSE  # Measure Offset
            w524 = T18 {"Time Stamp"=timestamp(0 s since 1904-01-01), "Results (Dictionary)"=[]}  # Results
            w531 = Status--enum."idle"  # DAQ Status
            # "starts in idle mode"
            # "Initialize the shift-register data, here.\n(data names are defined by what you wire into the bundle function)"
            n293 = local write "Status"(w531) -> ()
            n294 = call "DAQ.getDAQState.vi"("error in (no error)"=w528, "status"=w531, "Instrument.DAQ"=w527) -> ("error out"=w530:errorcluster)  [unwired: 7 in, 1 out]
            n295 = call <vilib>:"Add State(s) to Queue__jki_lib_state_machine.vi"("State(s) in (\"\")"=w535) -> ("States Out"=w534:string)  [unwired: 14 in]
            n296 = Bundle("Core"=w526, "SMO"=w527, "DAQ Status"=w531, "DAQmx Status"=w523, "Sweep Status"=w521, "Results"=w524, "SweepWaveforms"=w525, "Measure Offset"=w529, "Saved Amplitudes"=w522) -> (w532:T19)  [unwired: 1 in]
          }
          frame "Data: Process State" {
            # "Data: Process State.\n()"
            n297 = Unbundle By Name(w540) -> ("DAQmx Status"=w538:T2)
            n298 = case shown="\"clearing\"" w538 {
              tunnel: [Status--enum."idle" ("state") Status--enum."idle" ("state") Status--enum."idle" ("state") Status--enum."idle" ("state") Status--enum."created" ("state") Status--enum."created" ("state") Status--enum."started" ("state") Status--enum."started" ("state") Status--enum."stopped" ("state") Status--enum."idle" ("state") Status--enum."idle" ("state")] -> w536
              frame "idle", Default {
              }
              frame "calibrating" {
              }
              frame "configuring" {
              }
              frame "creating" {
              }
              frame "created" {
              }
              frame "starting" {
              }
              frame "started" {
              }
              frame "stopping" {
              }
              frame "stopped" {
              }
              frame "clearing" {
              }
              frame "error" {
              }
            }
            "Status" <- w536
            n299 = Unbundle By Name(w540) -> ("SMO"=w543:refnum<class "Instrument.DAQ.lvclass">)
            n300 = call "DAQ.getDAQState.vi"("error in (no error)"=w541, "status"=w536, "Instrument.DAQ"=w543) -> ("error out"=w537:errorcluster, "Instrument.DAQ out"=w539:refnum<class "Instrument.DAQ.lvclass">)  [unwired: 7 in]
            n301 = Bundle By Name(cluster=w540, "SMO"=w539, "DAQ Status"=w536) -> (w542:T19)
            n302 = call <vilib>:"Add State(s) to Queue__jki_lib_state_machine.vi"("State(s) in (\"\")"=w546) -> ("States Out"=w545:string)  [unwired: 14 in]
          }
          frame "Data: Process Devices" {
            # "Data: Process Devices.\n()"
            n303 = Unbundle By Name(w562) -> ("SMO"=w561:refnum<class "Instrument.DAQ.lvclass">)
            n304 = Unbundle By Name(w561) -> ("Devices"=w558:T65[])
            n305 = call "DAQ.getDeviceIDN.vi"("error in (no error)"=w559, "Devices"=w558, "Instrument.DAQ"=w561) -> ("error out"=w560:errorcluster, "Instrument.DAQ out"=w564:refnum<class "Instrument.DAQ.lvclass">)  [unwired: 7 in]
            n306 = Bundle By Name(cluster=w562, "SMO"=w564) -> (w563:T19)
            n307 = call <vilib>:"Add State(s) to Queue__jki_lib_state_machine.vi"("State(s) in (\"\")"=w567) -> ("States Out"=w566:string)  [unwired: 14 in]
          }
          frame "Data: Process Calibration" {
            # "Data: Process Calibration.\n()"
            n308 = Unbundle By Name(w568) -> ("SMO"=w572:refnum<class "Instrument.DAQ.lvclass">)
            n309 = Unbundle By Name(w572) -> ("Calibration"=w573:T66)
            n310 = call "DAQ.getCalibration.vi"("error in (no error)"=w570, "Calibration"=w573, "Instrument.DAQ"=w572) -> ("error out"=w571:errorcluster, "Instrument.DAQ"=w574:refnum<class "Instrument.DAQ.lvclass">)  [unwired: 7 in]
            n311 = Bundle By Name(cluster=w568, "SMO"=w574) -> (w569:T19)
            n312 = call <vilib>:"Add State(s) to Queue__jki_lib_state_machine.vi"("State(s) in (\"\")"=w577) -> ("States Out"=w576:string)  [unwired: 14 in]
          }
          frame "Data: Process DAQ" {
            # "Data: Process DAQ.\n()"
            n313 = Unbundle By Name(w589) -> ("SMO"=w587:refnum<class "Instrument.DAQ.lvclass">)
            n314 = Unbundle By Name(w587) -> ("DAQmx"=w585:refnum<class "DAQmx.lvclass">, "AI"=w583:T23, "AO"=w584:T20)
            n315 = call "config not UI to UI (AO and AI).vi"("error in (no error)"=w582, "AO Config"=w584, "AI Config"=w583) -> ("error out"=w581:errorcluster, "New Ch []"=w588:T67)  [unwired: 7 in]
            n316 = call "DAQ.getDAQconfig.vi"("error in (no error)"=w581, "New Ch []"=w588, "Instrument.DAQ"=w587) -> ("error out"=w580:errorcluster, "Instrument.DAQ out"=w586:refnum<class "Instrument.DAQ.lvclass">)  [unwired: 7 in]
            n317 = case shown="Default" w578 {
              tunnel: w585 -> [_ w601]
              tunnel: w584 -> [_ w599]
              tunnel: w583 -> [_ w598]
              tunnel: w580 -> [w594 w597]
              tunnel: [w594 w595] -> w579
              frame "-DAQmx" {
              }
              frame Default {
                n318 = call "setAIconfig.vi"("error in (no error)"=w597, "AIconfig"=w598, "DAQmx in"=w601) -> ("error out"=w596:errorcluster, "DAQmx out"=w600:refnum<class "DAQmx.lvclass">)  [unwired: 7 in]
                n319 = call "setAOconfig.vi"("error in (no error)"=w596, "AOconfig"=w599, "DAQmx in"=w600) -> ("error out"=w595:errorcluster)  [unwired: 7 in, 1 out]
              }
            }
            n320 = Bundle By Name(cluster=w589, "SMO"=w586) -> (w590:T19)
            n321 = call <vilib>:"Add State(s) to Queue__jki_lib_state_machine.vi"("State(s) in (\"\")"=w593) -> ("States Out"=w592:string)  [unwired: 14 in]
          }
          frame "Data: Process Sampling" {
            # "Data: Process Sampling.\n(Preprocess Sampling)"
            n322 = Unbundle By Name(w618) -> ("SMO"=w617:refnum<class "Instrument.DAQ.lvclass">)
            n323 = Unbundle By Name(w617) -> ("DSP"=w611:refnum<class "DSP.lvclass">, "Generator"=w606:refnum<class "Generator.lvclass">)
            n324 = Unbundle By Name(w617) -> ("DAQmx"=w616:refnum<class "DAQmx.lvclass">, "Sampling"=w602:T34)
            n325 = call "DAQ.getSampling.vi"("error in (no error)"=w608, "Sampling"=w602, "Instrument.DAQ"=w617) -> ("error out"=w610:errorcluster, "Instrument.DAQ out"=w613:refnum<class "Instrument.DAQ.lvclass">)  [unwired: 7 in]
            n326 = call "Write Timing.vi"("error in (no error)"=w610, "Timing"=w602, "DSP in"=w611) -> ("error out"=w609:errorcluster, "DSP out"=w614:refnum<class "DSP.lvclass">)  [unwired: 7 in]
            n327 = Bundle By Name(cluster=w613, "DSP"=w614) -> (w612:refnum<class "Instrument.DAQ.lvclass">)
            n328 = case shown="Default" w615 {
              tunnel: w616 -> [_ w627]
              tunnel: w602 -> [_ w626]
              tunnel: w609 -> [w623 w625]
              tunnel: [w623 w624] -> w605
              frame "-DAQmx" {
              }
              frame Default {
                n329 = call "setTiming.vi"("error in (no error)"=w625, "Timing"=w626, "DAQmx in"=w627) -> ("error out"=w624:errorcluster)  [unwired: 7 in, 1 out]
              }
            }
            n330 = Unbundle By Name(w602) -> ("Sampling"=w603:T35)
            n331 = call "setSampling.vi"("error in (no error)"=w605, "Sampling"=w603, "Generator in"=w606) -> ("error out"=w604:errorcluster)  [unwired: 7 in, 1 out]
            n332 = Bundle By Name(cluster=w618, "SMO"=w612) -> (w619:T19)
            n333 = call <vilib>:"Add State(s) to Queue__jki_lib_state_machine.vi"("State(s) in Front (\"\")"="" ("f"), "State(s) in (\"\")"=w622) -> ("States Out"=w621:string)  [unwired: 13 in]
          }
          frame "Data: Process AI Channels" {
            # "Data: Process AI Channels.\n()"
            n334 = Unbundle By Name(w639) -> ("SMO"=w638:refnum<class "Instrument.DAQ.lvclass">)
            n335 = call "Initialize AI Channels.vi"("error in (no error)"=w636, "Instrument.DAQ"=w638) -> ("error out"=w637:errorcluster, "Instrument.DAQ out"=w635:refnum<class "Instrument.DAQ.lvclass">)  [unwired: 8 in]
            n336 = Unbundle By Name(w635) -> ("Cfg_AI"=w628:T30)
            n337 = Unbundle By Name(w635) -> ("DSP"=w634:refnum<class "DSP.lvclass">)
            n338 = call "DAQ.getAIChannels.vi"("error in (no error)"=w637, "Channels.AI"=w628, "Instrument.DAQ"=w635) -> ("error out"=w632:errorcluster, "Instrument.DAQ out"=w630:refnum<class "Instrument.DAQ.lvclass">)  [unwired: 7 in]
            n339 = call "Write AI Channels.vi"("error in (no error)"=w632, "AI Channels"=w628, "DSP in"=w634) -> ("error out"=w631:errorcluster, "DSP out"=w633:refnum<class "DSP.lvclass">)  [unwired: 7 in]
            n340 = Bundle By Name(cluster=w630, "DSP"=w633) -> (w629:refnum<class "Instrument.DAQ.lvclass">)
            n341 = Bundle By Name(cluster=w639, "SMO"=w629) -> (w640:T19)
            n342 = call <vilib>:"Add State(s) to Queue__jki_lib_state_machine.vi"("State(s) in (\"\")"=w643) -> ("States Out"=w642:string)  [unwired: 14 in]
          }
          frame "Data: Process AO Channels" {
            # "Data: Process AO Channels.\n()"
            n343 = Unbundle By Name(w664) -> ("SMO"=w663:refnum<class "Instrument.DAQ.lvclass">)
            n344 = call "Initialize AO Channels.vi"("error in (no error)"=w662, "Instrument.DAQ"=w663) -> ("error out"=w656:errorcluster, "Instrument.DAQ out"=w661:refnum<class "Instrument.DAQ.lvclass">)  [unwired: 8 in]
            n345 = call "Limit AO Amplitude.vi"("error in (no error)"=w656, "Instrument.DAQ"=w661) -> ("error out"=w654:errorcluster, "Instrument.DAQ out"=w659:refnum<class "Instrument.DAQ.lvclass">)  [unwired: 8 in]
            n346 = call "Limit AO DC.vi"("error in (no error)"=w654, "Instrument.DAQ"=w659) -> ("error out"=w653:errorcluster, "Instrument.DAQ out"=w658:refnum<class "Instrument.DAQ.lvclass">)  [unwired: 8 in]
            n347 = call "Set all f same.vi"("error in (no error)"=w653, "Instrument.DAQ"=w658) -> ("error out"=w645:errorcluster, "Instrument.DAQ out"=w647:refnum<class "Instrument.DAQ.lvclass">)  [unwired: 8 in]
            n348 = Unbundle By Name(w647) -> ("Cfg_AO"=w657:T27)
            n349 = call "Divide Amplitude and Offset by Output Gain.vi"("error in (no error)"=w645, "Instrument.DAQ"=w647) -> ("error out"=w644:errorcluster, "Instrument.DAQ out"=w646:refnum<class "Instrument.DAQ.lvclass">)  [unwired: 8 in]
            n350 = call "Merge AO Settings to Generator.vi"("error in (no error)"=w644, "Instrument.DAQ in"=w646) -> ("error out"=w652:errorcluster, "AO Channels"=w648:T61, "Instrument.DAQ out"=w649:refnum<class "Instrument.DAQ.lvclass">)  [unwired: 7 in]
            n351 = Unbundle By Name(w649) -> ("Generator"=w650:refnum<class "Generator.lvclass">)
            n352 = call "setAOChannels.vi"("error in (no error)"=w652, "AO Channels"=w648, "Generator in"=w650) -> ("error out"=w651:errorcluster)  [unwired: 7 in, 1 out]
            n353 = call "DAQ.getAOChannels.vi"("error in (no error)"=w651, "Channels: AO"=w657, "Instrument.DAQ"=w647) -> ("error out"=w655:errorcluster, "Instrument.DAQ out"=w660:refnum<class "Instrument.DAQ.lvclass">)  [unwired: 7 in]
            n354 = Bundle By Name(cluster=w664, "SMO"=w660) -> (w665:T19)
            n355 = call <vilib>:"Add State(s) to Queue__jki_lib_state_machine.vi"("State(s) in (\"\")"=w668) -> ("States Out"=w667:string)  [unwired: 14 in]
          }
          frame "Data: Process REF Channels" {
            # "Data: Process REF Channels.\n()"
            n356 = Unbundle By Name(w684) -> ("SMO"=w682:refnum<class "Instrument.DAQ.lvclass">)
            n357 = call "Initialize REF Channels.vi"("error in (no error)"=w683, "Instrument.DAQ"=w682) -> ("error out"=w681:errorcluster, "Instrument.DAQ out"=w679:refnum<class "Instrument.DAQ.lvclass">)  [unwired: 8 in]
            n358 = call "Set all f same.vi"("error in (no error)"=w681, "Instrument.DAQ"=w679) -> ("error out"=w680:errorcluster, "Instrument.DAQ out"=w678:refnum<class "Instrument.DAQ.lvclass">)  [unwired: 8 in]
            n359 = Unbundle By Name(w678) -> ("Cfg_REF"=w672:T32)
            n360 = Unbundle By Name(w678) -> ("DSP"=w677:refnum<class "DSP.lvclass">, "Generator"=w671:refnum<class "Generator.lvclass">)
            n361 = call "DAQ.getREFChannels.vi"("error in (no error)"=w680, "Channels.REF"=w672, "Instrument.DAQ"=w678) -> ("error out"=w673:errorcluster, "Instrument.DAQ out"=w676:refnum<class "Instrument.DAQ.lvclass">)  [unwired: 7 in]
            n362 = call "Write REF Channels.vi"("error in (no error)"=w673, "REF Channels"=w672, "DSP in"=w677) -> ("error out"=w670:errorcluster, "DSP out"=w674:refnum<class "DSP.lvclass">)  [unwired: 7 in]
            n363 = Bundle By Name(cluster=w676, "DSP"=w674) -> (w675:refnum<class "Instrument.DAQ.lvclass">)
            n364 = call "setREFChannels.vi"("error in (no error)"=w670, "REF Channels"=w672, "Generator in"=w671) -> ("error out"=w669:errorcluster)  [unwired: 7 in, 1 out]
            n365 = Bundle By Name(cluster=w684, "SMO"=w675) -> (w685:T19)
            n366 = call <vilib>:"Add State(s) to Queue__jki_lib_state_machine.vi"("State(s) in (\"\")"=w688) -> ("States Out"=w687:string)  [unwired: 14 in]
          }
          frame "Data: Process Input Gain" {
            # "Do not put any code in this frame.\n(It is a separator no-op. You can make a copy of this frame to create a new Data frame)"
            n367 = Unbundle By Name(w695) -> ("SMO"=w697:refnum<class "Instrument.DAQ.lvclass">)
            n368 = call "Initialize Input Gain.vi"("error in (no error)"=w691, "Instrument.DAQ"=w697) -> ("error out"=w693:errorcluster, "Input Gain"=w689:T69, "Instrument.DAQ out"=w694:refnum<class "Instrument.DAQ.lvclass">)  [unwired: 7 in]
            n369 = call "DAQ.getInputGain.vi"("error in (no error)"=w693, "Input Gain"=w689, "Instrument.DAQ"=w694) -> ("error out"=w690:errorcluster, "Instrument.DAQ out"=w692:refnum<class "Instrument.DAQ.lvclass">)  [unwired: 7 in]
            n370 = Bundle By Name(cluster=w695, "SMO"=w692) -> (w696:T19)
            n371 = call <vilib>:"Add State(s) to Queue__jki_lib_state_machine.vi"("State(s) in (\"\")"=w700) -> ("States Out"=w699:string)  [unwired: 14 in]
          }
          frame "Data: Process Input Offset" {
            # "Do not put any code in this frame.\n(It is a separator no-op. You can make a copy of this frame to create a new Data frame)"
            n372 = Unbundle By Name(w708) -> ("SMO"=w705:refnum<class "Instrument.DAQ.lvclass">)
            n373 = call "Initialize Input Offset.vi"("error in (no error)"=w702, "Instrument.DAQ"=w705) -> ("error out"=w701:errorcluster, "Offset out"=w704:T69, "Instrument.DAQ out"=w703:refnum<class "Instrument.DAQ.lvclass">)  [unwired: 7 in]
            n374 = call "DAQ.getInputOffset.vi"("error in (no error)"=w701, "Input Offset"=w704, "Instrument.DAQ"=w703) -> ("error out"=w706:errorcluster, "Instrument.DAQ out"=w707:refnum<class "Instrument.DAQ.lvclass">)  [unwired: 7 in]
            n375 = Bundle By Name(cluster=w708, "SMO"=w707) -> (w709:T19)
            n376 = call <vilib>:"Add State(s) to Queue__jki_lib_state_machine.vi"("State(s) in (\"\")"=w712) -> ("States Out"=w711:string)  [unwired: 14 in]
          }
          frame "Data: Process Output Gain" {
            # "Do not put any code in this frame.\n(It is a separator no-op. You can make a copy of this frame to create a new Data frame)"
            n377 = Unbundle By Name(w719) -> ("SMO"=w721:refnum<class "Instrument.DAQ.lvclass">)
            n378 = call "Initialize Ouput Gain.vi"("error in (no error)"=w714, "Instrument.DAQ"=w721) -> ("error out"=w716:errorcluster, "Output Gain"=w713:T69, "Instrument.DAQ out"=w718:refnum<class "Instrument.DAQ.lvclass">)  [unwired: 7 in]
            n379 = call "DAQ.getOutputGain.vi"("error in (no error)"=w716, "Output Gain"=w713, "Instrument.DAQ"=w718) -> ("error out"=w715:errorcluster, "Instrument.DAQ out"=w717:refnum<class "Instrument.DAQ.lvclass">)  [unwired: 7 in]
            n380 = Bundle By Name(cluster=w719, "SMO"=w717) -> (w720:T19)
            n381 = call <vilib>:"Add State(s) to Queue__jki_lib_state_machine.vi"("State(s) in (\"\")"=w724) -> ("States Out"=w723:string)  [unwired: 14 in]
          }
          frame "Data: Process Sweep" {
            # "Do any necessary pre-processing here"
            # "Do not put any code in this frame.\n(It is a separator no-op. You can make a copy of this frame to create a new Data frame)"
            n382 = Unbundle By Name(w737) -> ("SMO"=w736:refnum<class "Instrument.DAQ.lvclass">)
            n383 = call "Initialize Sweep Channels.vi"("error in (no error)"=w735, "Instrument.DAQ"=w736) -> ("error out"=w728:errorcluster, "Instrument.DAQ out"=w729:refnum<class "Instrument.DAQ.lvclass">)  [unwired: 8 in]
            n384 = Unbundle By Name(w729) -> ("Sweep"=w730:T37)
            n385 = call "DAQ.getSweepChannels.vi"("error in (no error)"=w728, "Channels.Sweep"=w730, "Instrument.DAQ"=w729) -> ("error out"=w725:errorcluster, "Instrument.DAQ out"=w727:refnum<class "Instrument.DAQ.lvclass">)  [unwired: 7 in]
            n386 = Unbundle By Name(w727) -> ("Generator"=w733:refnum<class "Generator.lvclass">)
            n387 = call "Divide Sweep Config by Output Gain.vi"("error in (no error)"=w725, "Instrument.DAQ"=w727) -> ("error out"=w726:errorcluster, "Instrument.DAQ out"=w732:refnum<class "Instrument.DAQ.lvclass">)  [unwired: 8 in]
            n388 = Unbundle By Name(w732) -> ("Sweep"=w731:T37)
            n389 = call "setSweepChannels.vi"("error in (no error)"=w726, "Sweep Channels"=w731, "Generator in"=w733) -> ("error out"=w734:errorcluster)  [unwired: 7 in, 1 out]
            n390 = Bundle By Name(cluster=w737, "SMO"=w727) -> (w738:T19)
            n391 = call <vilib>:"Add State(s) to Queue__jki_lib_state_machine.vi"("State(s) in (\"\")"=w741) -> ("States Out"=w740:string)  [unwired: 14 in]
          }
          frame "Data: Update AO Channels" {
            n392 = Unbundle By Name(w746) -> ("SMO"=w745:refnum<class "Instrument.DAQ.lvclass">)
            n393 = Unbundle By Name(w745) -> ("Cfg_AO"=w747:T27)
            n394 = call "Is Value Changed.vim"("value"=w747) -> ("changed or first call?"=w744:bool)
            n395 = case shown="True" w744 {
              tunnel: w747 -> [_ w755]
              tunnel: w745 -> [_ w754]
              tunnel: [w751 w752] -> w743
              tunnel: w742 -> [w751 w753]
              frame False {
              }
              frame True {
                n396 = call "DAQ.getAOChannels.vi"("error in (no error)"=w753, "Channels: AO"=w755, "Instrument.DAQ"=w754) -> ("error out"=w752:errorcluster)  [unwired: 7 in, 1 out]
              }
            }
            n397 = call <vilib>:"Add State(s) to Queue__jki_lib_state_machine.vi"("State(s) in (\"\")"=w750) -> ("States Out"=w749:string)  [unwired: 14 in]
          }
          frame "Data: Zero Amplitude" {
            n398 = Unbundle By Name(w759) -> ("SMO"=w762:refnum<class "Instrument.DAQ.lvclass">)
            n399 = call "Zero AO Amplitudes.vi"("error in (no error)"=w757, "Instrument.DAQ in"=w762) -> ("error out"=w758:errorcluster, "Saved Amplitudes"=w756:dbl[], "Instrument.DAQ out"=w761:refnum<class "Instrument.DAQ.lvclass">)  [unwired: 7 in]
            n400 = Bundle By Name(cluster=w759, "SMO"=w761, "Saved Amplitudes"=w756) -> (w760:T19)
            n401 = call <vilib>:"Add State(s) to Queue__jki_lib_state_machine.vi"("State(s) in (\"\")"=w765) -> ("States Out"=w764:string)  [unwired: 14 in]
          }
          frame "Data: Restore Amplitude" {
            n402 = Unbundle By Name(w771) -> ("SMO"=w767:refnum<class "Instrument.DAQ.lvclass">, "Saved Amplitudes"=w770:dbl[])
            n403 = call "Restore AO Amplitudes.vi"("error in (no error)"=w769, "Saved Amplitudes"=w770, "Instrument.DAQ in"=w767) -> ("error out"=w768:errorcluster, "Instrument.DAQ out"=w766:refnum<class "Instrument.DAQ.lvclass">)  [unwired: 7 in]
            n404 = Bundle By Name(cluster=w771, "SMO"=w766) -> (w772:T19)
            n405 = call <vilib>:"Add State(s) to Queue__jki_lib_state_machine.vi"("State(s) in (\"\")"=w775) -> ("States Out"=w774:string)  [unwired: 14 in]
          }
          frame "Data: Clear Sweep Data" {
            w778 = waveform(dbl)[] [] ("X")
            n406 = Unbundle By Name(w783) -> ("SMO"=w782:refnum<class "Instrument.DAQ.lvclass">)
            n407 = Bundle By Name(cluster=T11 {"AO"=[], "AI"=[], "X"=[], "Y"=[]} ("SweepWFMs"), "AO"=w778, "AI"=w778, "X"=w778, "Y"=w778) -> (w776:T11)
            n408 = call "DAQ.getSweepWaveforms.vi"("error in (no error)"=w781, "SweepWFMs"=w776, "Instrument.DAQ"=w782) -> ("error out"=w779:errorcluster, "Instrument.DAQ out"=w780:refnum<class "Instrument.DAQ.lvclass">)  [unwired: 7 in]
            n409 = Bundle By Name(cluster=w783, "SMO"=w780, "SweepWaveforms"=w776) -> (w784:T19)
            n410 = call <vilib>:"Add State(s) to Queue__jki_lib_state_machine.vi"("State(s) in (\"\")"=w787) -> ("States Out"=w786:string)  [unwired: 14 in]
          }
          frame "Data: Save Sweep Data" {
            # "publish intermediate waveform"
            n411 = Unbundle By Name(w807) -> ("SweepWaveforms"=w805:T11)
            n412 = Unbundle By Name(w807) -> ("SMO"=w800:refnum<class "Instrument.DAQ.lvclass">)
            n413 = Unbundle By Name(w800) -> ("AO"=w804:waveform(dbl)[], "AI"=w803:waveform(dbl)[], "X"=w802:waveform(dbl)[], "Y"=w801:waveform(dbl)[])
            n414 = flat-sequence {
              tunnel: [w823] -> w793
              tunnel: w798 -> [w822]
              tunnel: [w822] -> w794
              frame #0 {
                n415 = call <vilib>:"High Resolution Relative Seconds.vi"() -> ("relative seconds"=w823:dbl)
              }
            }
            n416 = Bundle By Name(cluster=T11 {"AO"=[], "AI"=[], "X"=[], "Y"=[]} ("SweepWFMs"), "AO"=w804, "AI"=w803, "X"=w802, "Y"=w801) -> (w799:T11)
            n417 = call "DAQ.getSweepWaveforms.vi"("error in (no error)"=w794, "SweepWFMs"=w799, "Instrument.DAQ"=w800) -> ("Instrument.DAQ out"=w792:refnum<class "Instrument.DAQ.lvclass">)  [unwired: 7 in, 1 out]
            n418 = call "Append Sweep Waveforms.vi"("error in (no error)"=w794, "New SweepWaveforms"=w799, "SweepWaveforms in"=w805) -> ("error out"=w790:errorcluster, "SweepWaveforms out"=w788:T11)  [unwired: 7 in]
            n419 = case shown="\"final\"" w789 {
              tunnel: w792 -> [_ w817]
              tunnel: w788 -> [_ w816]
              tunnel: [w812 w819] -> w791
              tunnel: w790 -> [w812 w814]
              frame Default {
              }
              frame "final" {
                n420 = call "DAQ.getDAQState.vi"("error in (no error)"=w814, "status"=Status--enum."started", "Instrument.DAQ"=w817) -> ("error out"=w815:errorcluster, "Instrument.DAQ out"=w818:refnum<class "Instrument.DAQ.lvclass">)  [unwired: 7 in]
                n421 = call "DAQ.getSweepWaveforms.vi"("error in (no error)"=w815, "SweepWFMs"=w816, "Instrument.DAQ"=w818) -> ("error out"=w819:errorcluster)  [unwired: 7 in, 1 out]
              }
            }
            n422 = Bundle By Name(cluster=w807, "SweepWaveforms"=w788) -> (w808:T19)
            n423 = flat-sequence {
              tunnel: [w821] -> w796
              tunnel: w791 -> [w820]
              tunnel: [w820] -> w797
              frame #0 {
                n424 = call <vilib>:"High Resolution Relative Seconds.vi"() -> ("relative seconds"=w821:dbl)
              }
            }
            n425 = Subtract(x=w796, y=w793) -> (x-y=→"Sweep Chart":dbl)
            n426 = call <vilib>:"Add State(s) to Queue__jki_lib_state_machine.vi"("State(s) in (\"\")"=w811) -> ("States Out"=w810:string)  [unwired: 14 in]
          }
          frame "Data: Save Intermediate Sweep Data" {
            n427 = call <userlib>:"Periodic Trigger__ogtk.vi"("time (ms)"=u32 1000) -> ()  [unwired: 12 in, 3 out]
            n428 = case shown="True" FALSE {
              tunnel: [w833 w839] -> w829
              tunnel: w828 -> [w833 w838]
              tunnel: [w834 w836] -> w827
              tunnel: w826 -> [w834 w835]
              frame False {
              }
              frame True {
                # "periodically publish waveform and clear buffer:\n- save sooner and more often\n- enable longer sweeps\n#todo\nchange to or add buffer for lossless logging"
                n429 = Unbundle By Name(w835) -> ("SMO"=w841:refnum<class "Instrument.DAQ.lvclass">, "SweepWaveforms"=w840:T11)
                n430 = call "DAQ.getSweepWaveforms.vi"("error in (no error)"=w838, "SweepWFMs"=w840, "Instrument.DAQ"=w841) -> ("error out"=w839:errorcluster)  [unwired: 7 in, 1 out]
                n431 = Bundle By Name(cluster=w835, "SweepWaveforms"=T11 {"AO"=[], "AI"=[], "X"=[], "Y"=[]}) -> (w836:T19)
              }
            }
            n432 = call <vilib>:"Add State(s) to Queue__jki_lib_state_machine.vi"("State(s) in (\"\")"=w832) -> ("States Out"=w831:string)  [unwired: 14 in]
          }
          frame "Data: Cleanup" {
            # "Cleanup any data and references, here.\n(this is called automatically, by the Macro: Exit)"
            n433 = Unbundle By Name(w842) -> ("Core.Current VI Reference"=w846:refnum<vi>)
            n434 = Close Reference(reference=w846, error in (no error)=w845) -> (error out=w844:errorcluster)
            n435 = call <vilib>:"Add State(s) to Queue__jki_lib_state_machine.vi"("State(s) in (\"\")"=w848) -> ("States Out"=w847:string)  [unwired: 14 in]
          }
          frame "---------- UI ----------" {
            # "Do not put any code in this frame.\n(It is a separator no-op. You can make a copy of this frame to create a new UI frame)"
            n436 = call <vilib>:"Add State(s) to Queue__jki_lib_state_machine.vi"("State(s) in (\"\")"=w853) -> ("States Out"=w852:string)  [unwired: 14 in]
          }
          frame "UI: Initialize" {
            # "Initialize the User Interface, here.\n(this is called automatically, by the Macro: Init)"
            n437 = call <userlib>:"Fit VI window to Largest Dec__ogtk.vi"("error in (no error)"=w856, "border spacing (2 px)"=0) -> ("error out"=w857:errorcluster)  [unwired: 4 in, 1 out]
            n438 = local write "Tab Control"(enum32{"Default", "Advanced"}."Default" ("Tab Control")) -> ()
            n439 = local write "Method"("" ("String")) -> ()
            n440 = call <vilib>:"Add State(s) to Queue__jki_lib_state_machine.vi"("State(s) in (\"\")"=w862) -> ("States Out"=w861:string)  [unwired: 14 in]
          }
          frame "UI: Wait" {
            # "UI: Wait.\n(use: \"UI: Wait >> time\" (in ms))"
            n441 = Scan From String(format string="%d", input string=w863, default 1=u32 0 ("default value 1")) -> (output 1=w871:u32)  [unwired: 2 in, 3 out]
            n442 = feedback #1(TRUE ("Triggered")) -> (w868:bool)
            n443 = call <userlib>:"Periodic Trigger__ogtk.vi"("time (ms)"=w871, "reset"=w868) -> ("Triggered"=w869:bool)  [unwired: 11 in, 2 out]
            n444 = feedback-in #1(w869) -> ()
            n445 = call <vilib>:"Build State String with Arguments__JKI_lib_State_Machine.vi"("Arguments (\"\")"=w863, "State"=w867) -> ("State with Arguments"=w866:string)  [unwired: 4 in]
            n446 = Select(t="", s=w869, f=w866) -> (s? t:f=w864:string)
            n447 = call <vilib>:"Add State(s) to Queue__jki_lib_state_machine.vi"("State(s) in Front (\"\")"=w864, "State(s) in (\"\")"=w878) -> ("States Out"=w877:string)  [unwired: 13 in]
          }
          frame "UI: Cursor Set" {
            # "Argument"
            # "Initialize the User Interface, here.\n(this is called automatically, by the Macro: Init)"
            n448 = disable-structure shown="Default" {
              disable-tunnel: w881 -> [w886 w889]
              disable-tunnel: [w886 w888] -> w880
              disable-tunnel: w879 -> [_ w887]
              frame condition #0 {
              }
              frame condition #1 (active) {
                n449 = case shown="\"Idle\", Default" w887 {
                  tunnel: w889 -> [w891 w893]
                  tunnel: [w890 w892] -> w888
                  frame "Idle", Default {
                    n450 = call <vilib>:"Unset Busy.vi"("error in (no error)"=w891) -> ("error out"=w890:errorcluster)  [unwired: 10 in]
                  }
                  frame "Busy" {
                    n451 = call <vilib>:"Set Busy.vi"("error in (no error)"=w893) -> ("error out"=w892:errorcluster)  [unwired: 9 in, 1 out]
                  }
                }
              }
            }
            n452 = call <vilib>:"Add State(s) to Queue__jki_lib_state_machine.vi"("State(s) in (\"\")"=w885) -> ("States Out"=w884:string)  [unwired: 14 in]
          }
          frame "UI: Front Panel State" {
            # "Argument"
            # "Set Front Panel Open or Closed\n(Usage: \"UI: Front Panel State >> Open|Close\")"
            n453 = Unbundle By Name(w897) -> ("Core.Current VI Reference"=w896:refnum<vi>)
            n454 = disable-structure shown="Default" {
              disable-tunnel: w899 -> [w905 w928]
              disable-tunnel: [w904 w928] -> w898
              disable-tunnel: w896 -> [w903 _]
              disable-tunnel: w895 -> [w902 _]
              frame condition #0 (active) {
                n455 = case shown="\"Close\"" w902 {
                  tunnel: w905 -> [w909 w922]
                  tunnel: [w911 w923] -> w904
                  tunnel: w903 -> [w910 w920]
                  frame "Open", Default {
                    n456 = property class="VI"(reference=w910, error in=w909) -> (reference out=w907:refnum<vi>, error out=w908:errorcluster, "FP.State"=w906:T12)
                    n457 = case shown="\"Closed\"" w906 {
                      tunnel: [w914 w917] -> w911
                      tunnel: w908 -> [w913 w917]
                      tunnel: w907 -> [w912 _]
                      frame "Closed" {
                        n458 = invoke class="VI" method="FP.Open"(reference=w912, error in=w913, "Activate"=TRUE, "State"=T12."Standard") -> (error out=w914:errorcluster)  [unwired: 1 in, 4 out]
                      }
                      frame Default {
                      }
                    }
                  }
                  frame "Close" {
                    n459 = property class="VI"(reference=w920, error in=w922) -> (reference out=w919:refnum<vi>, error out=w921:errorcluster, "FP.State"=w918:T12)
                    n460 = case shown="Default" w918 {
                      tunnel: [w924 w927] -> w923
                      tunnel: w921 -> [w924 w926]
                      tunnel: w919 -> [_ w925]
                      frame "Invalid", "Closed" {
                      }
                      frame Default {
                        n461 = invoke class="VI" method="FP.Close"(reference=w925, error in=w926) -> (error out=w927:errorcluster)  [unwired: 1 in, 2 out]
                      }
                    }
                  }
                }
              }
              frame condition #1 {
              }
            }
            n462 = call <vilib>:"Add State(s) to Queue__jki_lib_state_machine.vi"("State(s) in (\"\")"=w901) -> ("States Out"=w900:string)  [unwired: 14 in]
          }
          frame "---------- Macro ----------" {
            # "Do not put any code in this frame.\n(It is a separator no-op. You can make a copy of this frame to create a new Macro frame)"
            n463 = call <vilib>:"Add State(s) to Queue__jki_lib_state_machine.vi"("State(s) in (\"\")"=w933) -> ("States Out"=w932:string)  [unwired: 14 in]
          }
          frame "Macro: Initialize" {
            w936 = "UI: Initialize\nUI: Front Panel State >> Close\nMacro: Debug"  # UI: Initialize UI: Front Panel State >> Close Macro: Debug
            # "Initialization Macro\n(This is called once, when the VI starts)"
            n464 = call <vilib>:"Add State(s) to Queue__jki_lib_state_machine.vi"("State(s) in Front (\"\")"="Data: Initialize\nInitialize Core Data\nEvents: Register", "State(s) in (\"\")"="Process: Sync", "State(s) at Back (\"\")"=w936) -> ("States Out"=w935:string)  [unwired: 12 in]
            n465 = call <vilib>:"Add State(s) to Queue__jki_lib_state_machine.vi"("State(s) in Front (\"\")"=w935, "State(s) in (\"\")"=w942) -> ("States Out"=w941:string)  [unwired: 13 in]
          }
          frame "Macro: Debug" {
            # "exe?"
            # "If pane is an EXE, then close it when we exit"
            # "Macro: Debug\n(get debug behavior, determine UI and determine shutdown behavior)"
            n466 = Unbundle By Name(w945) -> ("Core.Close Panel on Exit?"=w949:bool, "SMO"=w954:refnum<class "Instrument.DAQ.lvclass">)
            n467 = property class="App"() -> ("App.Kind"=w952:T10)  [unwired: 2 in, 2 out]
            n468 = Equal?(x=w952, y=T10."Run Time System" ("Application:Kind")) -> (x = y?=w948:bool)
            n469 = call <userlib>:"Get Debug Mode.vi"("error in (no error)"=w943, "SMO"=w954) -> ("error out"=w944:errorcluster, "Behavior"=w953:T70)  [unwired: 7 in, 1 out]
            n470 = case shown="\"Normal\", Default" w953 {
              tunnel: [w958 w960] -> w950
              tunnel: w949 -> [w958 _]
              tunnel: w948 -> [_ w962]
              tunnel: [_ "UI: Front Panel State >> Open\nUI: Wait >> 1000"] -> w946
              frame "Normal", Default {
                # "respect core.close"
              }
              frame "Debug" {
                # "keep panel open\nunless exe"
                n471 = Or(x=w962, y=FALSE) -> (x .or. y?=w960:bool)
              }
            }
            n472 = Bundle By Name(cluster=w945, "Core.Close Panel on Exit?"=w950) -> (w947:T19)
            n473 = call <vilib>:"Add State(s) to Queue__jki_lib_state_machine.vi"("State(s) in Front (\"\")"=w946, "State(s) in (\"\")"=w957) -> ("States Out"=w956:string)  [unwired: 13 in]
          }
          frame "Macro: Post Error Handling" {
            # "Clear Last Error?"
            # "Handle any errors here.\nYou can also output any states to clean-up after errors occur"
            n474 = Unbundle By Name(w965) -> ("Core.Last Error.error"=w964:errorcluster, "Core.Last Error.remaining states"=w968:string, "Core.Shutdown?"=w969:bool, "SMO"=w963:refnum<class "Instrument.DAQ.lvclass">)
            n475 = Unbundle By Name(w965) -> ("Core.Last Error.error"=w972:errorcluster)
            n476 = case shown="True" FALSE {
              tunnel: w972 -> [w993 _]
              tunnel: [w993 _] -> w971
              frame False {
              }
              frame True {
              }
            }
            n477 = case shown="False" w969 {
              tunnel: w968 -> [_ w992]
              tunnel: [w978 w991] -> w967
              tunnel: w964 -> [w979 _]
              tunnel: w963 -> [w977 _]
              frame False {
                # "These are the remaining states (at the moment the error occured). States can be altered according to business logic."
                # "NOT SHUTTING DOWN"
                n478 = while {
                  tunnel: w979 -> [w985]
                  shift-right: [w985] -> _
                  shift-left: _ -> [w989]
                  tunnel: [w980] -> w978
                  tunnel: w977 -> [w984]
                  stop <- TRUE stop-if-true
                  n479 = Equal?(x=w989, y=w985) -> (x = y?=w986:bool)
                  n480 = call "DAQ.ErrorHandler.vi"("error in (no error)"=w985, "Lockin.DAQ in"=w984) -> ("DAQmx Error?"=w983:bool)  [unwired: 6 in, 3 out]
                  n481 = Select(t="DAQ: STOP", s=w986, f="Idle" ("States Out")) -> (s? t:f=w981:string)
                  n482 = Select(t=w981, s=w983, f="") -> (s? t:f=w980:string)
                }
              }
              frame True {
                # "Developer can decide to alter the states but should be aware that during the shutdown process, there are certain states that must be run for the SMO to properly shut itself (and this process) down. As such, one can add states to perform additional clean-ups, but should append the remaining state to be executed."
                # "SHUTTING DOWN"
                n483 = call <vilib>:"Add State(s) to Queue__jki_lib_state_machine.vi"("State(s) in (\"\")"=w992) -> ("States Out"=w991:string)  [unwired: 14 in]
              }
            }
            n484 = Bundle By Name(cluster=w965, "Core.Last Error.error"=w971) -> (w966:T19)
            n485 = call <vilib>:"Add State(s) to Queue__jki_lib_state_machine.vi"("State(s) in Front (\"\")"=w967, "State(s) in (\"\")"=w976) -> ("States Out"=w975:string)  [unwired: 13 in]
          }
          frame "Macro: Exit" {
            # "Exit Macro\n(This is called once, when the VI exits)"
            n486 = Unbundle By Name(w994) -> ("Core.Close Panel on Exit?"=w1007:bool)
            n487 = Bundle By Name(cluster=w994, "Core.Shutdown?"=TRUE) -> (w995:T19)
            n488 = Select(t="UI: Front Panel State >> Close", s=w1007, f="") -> (s? t:f=w1004:string)
            n489 = call <vilib>:"Add State(s) to Queue__jki_lib_state_machine.vi"("State(s) in Front (\"\")"="Data: Cleanup\nEvents: Unregister", "State(s) in (\"\")"="Process: Sync", "State(s) at Back (\"\")"="Exit") -> ("States Out"=w1001:string)  [unwired: 12 in]
            n490 = call <vilib>:"Add State(s) to Queue__jki_lib_state_machine.vi"("State(s) in Front (\"\")"="Macro: Stop DAQmx", "State(s) in (\"\")"=w1004, "State(s) at Back (\"\")"=w1001) -> ("States Out"=w999:string)  [unwired: 12 in]
            n491 = call <vilib>:"Add State(s) to Queue__jki_lib_state_machine.vi"("State(s) in Front (\"\")"=w999, "State(s) in (\"\")"=w1010) -> ("States Out"=w1009:string)  [unwired: 13 in]
          }
          frame "Macro: Start DAQmx" {
            # "Macro: Start.\n(checks the status of DAQmx process)"
            n492 = Unbundle By Name(w1012) -> ("DAQmx Status"=w1011:T2)
            n493 = case shown="\"creating\"" w1011 {
              tunnel: ["DAQ: START" ("State(s) in Front (\"\")") "" ("State(s) in Front (\"\")") "" ("State(s) in Front (\"\")") "idle\nMacro: Start DAQmx" ("State(s) in Front (\"\")") "DAQ: START" ("State(s) in Front (\"\")") "" ("State(s) in Front (\"\")") "" ("State(s) in Front (\"\")") "idle\nMacro: Start DAQmx" ("State(s) in Front (\"\")") "idle\nMacro: Start DAQmx" ("State(s) in Front (\"\")") "idle\nMacro: Start DAQmx" ("State(s) in Front (\"\")")] -> w1013
              frame "idle", Default {
              }
              frame "calibrating" {
              }
              frame "configuring" {
              }
              frame "creating" {
              }
              frame "created" {
              }
              frame "starting" {
              }
              frame "started" {
              }
              frame "stopping" {
              }
              frame "stopped" {
              }
              frame "clearing" {
              }
            }
            n494 = call <vilib>:"Add State(s) to Queue__jki_lib_state_machine.vi"("State(s) in Front (\"\")"=w1013, "State(s) in (\"\")"=w1017) -> ("States Out"=w1016:string)  [unwired: 13 in]
          }
          frame "Macro: Stop DAQmx" {
            # "Macro: Stop.\n(checks the status of DAQmx process)"
            n495 = Unbundle By Name(w1028) -> ("DAQmx Status"=w1030:T2)
            n496 = case shown="\"stopping\"" w1030 {
              tunnel: ["" ("State(s) in Front (\"\")") "" ("State(s) in Front (\"\")") "" ("State(s) in Front (\"\")") "idle\nMacro: Stop DAQmx" ("State(s) in Front (\"\")") "DAQ: STOP" ("State(s) in Front (\"\")") "idle\nMacro: Stop DAQmx" ("State(s) in Front (\"\")") "DAQ: STOP" ("State(s) in Front (\"\")") "" ("State(s) in Front (\"\")") "" ("State(s) in Front (\"\")") "" ("State(s) in Front (\"\")")] -> w1029
              frame "idle", Default {
              }
              frame "calibrating" {
              }
              frame "configuring" {
              }
              frame "creating" {
              }
              frame "created" {
              }
              frame "starting" {
              }
              frame "started" {
              }
              frame "stopping" {
              }
              frame "stopped" {
              }
              frame "clearing" {
              }
            }
            n497 = call <vilib>:"Add State(s) to Queue__jki_lib_state_machine.vi"("State(s) in Front (\"\")"=w1029, "State(s) in (\"\")"=w1034) -> ("States Out"=w1031:string)  [unwired: 13 in]
          }
          frame "Macro: DSP" {
            # "Macro: DSP.\n()"
            n498 = Unbundle By Name(w1054) -> ("SMO"=w1053:refnum<class "Instrument.DAQ.lvclass">)
            n499 = Unbundle By Name(w1053) -> ("AO"=w1046:waveform(dbl)[])
            n500 = call "Get Waveform Sweep Status.vi"("error in (no error)"=w1049, "Waveforms in"=w1046) -> ("error out"=w1050:errorcluster, "sweep status"=w1060:T13)  [unwired: 7 in, 1 out]
            n501 = Equal?(x=w1060, y=Generator.Sweep_Status--enum."sweeping" ("sweep status")) -> (x = y?=w1058:bool)
            n502 = call <userlib>:"Boolean Trigger__ogtk.vi"("Boolean Input"=w1058) -> ("Falling Edge"=w1055:bool)  [unwired: 1 in, 1 out]
            n503 = Select(t="Data: Save Sweep Data" ("State(s) at Back (\"\")"), s=w1058, f="") -> (s? t:f=w1052:string)
            n504 = Select(t="Data: Save Sweep Data >> final" ("State(s) at Back (\"\")"), s=w1055, f="") -> (s? t:f=w1051:string)
            n505 = call <vilib>:"Add State(s) to Queue__jki_lib_state_machine.vi"("State(s) in Front (\"\")"="DSP: Simulate\nDSP: Phase\nDSP: Filter\nDSP: Lockin" ("State(s) in Front (\"\")"), "State(s) in (\"\")"=w1052, "State(s) at Back (\"\")"=w1051) -> ("States Out"=w1047:string)  [unwired: 12 in]
            n506 = call <vilib>:"Add State(s) to Queue__jki_lib_state_machine.vi"("State(s) in Front (\"\")"=w1047, "State(s) in (\"\")"=w1064) -> ("States Out"=w1063:string)  [unwired: 13 in]
          }
          frame "---------- Process ----------" {
            # "Template Separator\n(You can make a copy of, or modify, this frame)"
            n507 = call <vilib>:"Add State(s) to Queue__jki_lib_state_machine.vi"("State(s) in (\"\")"=w1069) -> ("States Out"=w1068:string)  [unwired: 14 in]
          }
          frame "Process: Sync" {
            n508 = Unbundle By Name(w1077) -> ("SMO"=w1073:refnum<class "Instrument.DAQ.lvclass">)
            n509 = call <vilib>:"WaitOnProcessSync.vi"("error in (no error)"=w1072, "SMO"=w1073) -> ("error out"=w1071:errorcluster, "Don't run?"=w1076:bool)  [unwired: 7 in, 1 out]
            n510 = Select(t="Data: Cleanup\nEvents: Unregister\nExit", s=w1076, f="") -> (s? t:f=w1070:string)
            n511 = call <vilib>:"Add State(s) to Queue__jki_lib_state_machine.vi"("State(s) in Front (\"\")"=w1070, "State(s) in (\"\")"=w1080) -> ("States Out"=w1079:string)  [unwired: 13 in]
          }
          frame "---------- Events ----------" {
            # "Template Separator\n(You can make a copy of, or modify, this frame)"
            n512 = call <vilib>:"Add State(s) to Queue__jki_lib_state_machine.vi"("State(s) in (\"\")"=w1085) -> ("States Out"=w1084:string)  [unwired: 14 in]
          }
          frame "Events: Register" {
            n513 = Unbundle By Name(w1103) -> ("SMO"=w1102:refnum<class "Instrument.DAQ.lvclass">)
            n514 = call <vilib>:"GetProtectedEvents.vi"("SMO"=w1102) -> ("error out"=w1100:errorcluster, "SMO Protected Events"=w1099:T71, "SMO out"=w1094:refnum<class "Instrument.DAQ.lvclass">)  [unwired: 8 in]
            n515 = call "DAQ.GetPrivateEvents.vi"("Instrument.DAQ"=w1094) -> ("error out"=w1098:errorcluster, "DAQ Private Events"=w1093:T72, "Instrument.DAQ"=w1096:refnum<class "Instrument.DAQ.lvclass">)  [unwired: 8 in]
            n516 = Unbundle By Name(w1096) -> ("DAQmx"=w1092:refnum<class "DAQmx.lvclass">, "Generator"=w1091:refnum<class "Generator.lvclass">)
            n517 = call "DAQmx.GetPublicEvents.vi"("DAQmx"=w1092) -> ("error out"=w1095:errorcluster, "DAQmx Public Events"=w1086:T73)  [unwired: 8 in, 1 out]
            n518 = call "Generator.GetPublicEvents.vi"("Generator"=w1091) -> ("error out"=w1089:errorcluster, "Generator Public Events"=w1090:T74)  [unwired: 8 in, 1 out]
            n519 = register-events(w1099, w1093, w1086, w1090) -> (reference out=w1097:refnum<event-registration>, error out=w1087:errorcluster)  [unwired: 2 in]
            n520 = Merge Errors(w1088, w1087, w1089, w1095, w1098, w1100) -> (w1101:errorcluster)
            n521 = call <vilib>:"Add State(s) to Queue__jki_lib_state_machine.vi"("State(s) in (\"\")"=w1105) -> ("States Out"=w1104:string)  [unwired: 14 in]
          }
          frame "Events: Unregister" {
            n522 = Unregister For Events(event registration refnum=w1106, error in=w1108) -> (error out=w1107:errorcluster)
            n523 = call <vilib>:"Clear Errors.vi"("error in (no error)"=w1107) -> ()  [unwired: 5 in, 2 out]
            n524 = call <vilib>:"Add State(s) to Queue__jki_lib_state_machine.vi"("State(s) in (\"\")"=w1111) -> ("States Out"=w1110:string)  [unwired: 14 in]
          }
          frame "---------- DAQ ----------" {
            n525 = call <vilib>:"Add State(s) to Queue__jki_lib_state_machine.vi"("State(s) in (\"\")"=w1116) -> ("States Out"=w1115:string)  [unwired: 14 in]
          }
          frame "DAQ: AUTO" {
            n526 = Unbundle By Name(w1120) -> ("SMO"=w1122:refnum<class "Instrument.DAQ.lvclass">)
            n527 = call "DAQ.Auto Configure.vi"("error in (no error)"=w1121, "Instrument.DAQ"=w1122) -> ("error out"=w1117:errorcluster, "Instrument.DAQ out"=w1118:refnum<class "Instrument.DAQ.lvclass">)  [unwired: 8 in]
            n528 = Bundle By Name(cluster=w1120, "SMO"=w1118) -> (w1119:T19)
            n529 = call <vilib>:"Add State(s) to Queue__jki_lib_state_machine.vi"("State(s) in (\"\")"=w1125) -> ("States Out"=w1124:string)  [unwired: 14 in]
          }
          frame "DAQ: START" {
            n530 = Unbundle By Name(w1131) -> ("SMO"=w1129:refnum<class "Instrument.DAQ.lvclass">)
            n531 = call "DAQ.Start.vi"("error in"=w1126, "Instrument.DAQ"=w1129) -> ("error out"=w1127:errorcluster, "Instrument.DAQ out"=w1128:refnum<class "Instrument.DAQ.lvclass">)  [unwired: 8 in]
            n532 = Bundle By Name(cluster=w1131, "SMO"=w1128) -> (w1130:T19)
            n533 = call <vilib>:"Add State(s) to Queue__jki_lib_state_machine.vi"("State(s) in (\"\")"=w1134) -> ("States Out"=w1133:string)  [unwired: 14 in]
          }
          frame "DAQ: CALIBRATE" {
            # "calibrate or get calibration"
            n534 = Unbundle By Name(w1144) -> ("SMO"=w1142:refnum<class "Instrument.DAQ.lvclass">)
            n535 = Scan From String(input string=w1136, default 1=PrivateEvents--DAQ.setCalibration."Check" ("setCalibration")) -> (error out=w1135:errorcluster, output 1=w1137:T14)  [unwired: 3 in, 2 out]
            n536 = call <vilib>:"Clear Errors.vi"("error in (no error)"=w1135) -> ()  [unwired: 5 in, 2 out]
            n537 = case shown="\"Calibrate\"" w1137 {
              tunnel: w1142 -> [w1151 w1155]
              tunnel: [w1150 w1154] -> w1139
              tunnel: w1141 -> [w1148 w1153]
              tunnel: [w1149 w1152] -> w1140
              frame "Check" {
                n538 = call "DAQ.Get Calibration.vi"("error in (no error)"=w1148, "Instrument.DAQ in"=w1151) -> ("error out"=w1149:errorcluster, "Instrument.DAQ out"=w1150:refnum<class "Instrument.DAQ.lvclass">)  [unwired: 8 in]
              }
              frame "Calibrate" {
                n539 = call "DAQ.Calibrate.vi"("error in (no error)"=w1153, "Lockin.DAQ in"=w1155) -> ("error out"=w1152:errorcluster, "Lockin.DAQ out"=w1154:refnum<class "Instrument.DAQ.lvclass">)  [unwired: 8 in]
              }
            }
            n540 = Bundle By Name(cluster=w1144, "SMO"=w1139) -> (w1143:T19)
            n541 = call <vilib>:"Add State(s) to Queue__jki_lib_state_machine.vi"("State(s) in (\"\")"=w1147) -> ("States Out"=w1146:string)  [unwired: 14 in]
          }
          frame "DAQ: STOP" {
            n542 = Unbundle By Name(w1161) -> ("SMO"=w1159:refnum<class "Instrument.DAQ.lvclass">)
            n543 = call "DAQ.Stop.vi"("error in (no error)"=w1157, "Instrument.DAQ in"=w1159) -> ("error out"=w1156:errorcluster, "Instrument.DAQ out"=w1158:refnum<class "Instrument.DAQ.lvclass">)  [unwired: 8 in]
            n544 = Bundle By Name(cluster=w1161, "SMO"=w1158) -> (w1160:T19)
            n545 = call <vilib>:"Add State(s) to Queue__jki_lib_state_machine.vi"("State(s) in (\"\")"=w1164) -> ("States Out"=w1163:string)  [unwired: 14 in]
          }
          frame "---------- DSP ----------" {
            n546 = call <vilib>:"Add State(s) to Queue__jki_lib_state_machine.vi"("State(s) in (\"\")"=w1169) -> ("States Out"=w1168:string)  [unwired: 14 in]
          }
          frame "DSP: Simulate" {
            n547 = Unbundle By Name(w1172) -> ("SMO"=w1176:refnum<class "Instrument.DAQ.lvclass">)
            n548 = call "DAQ.Simulate Noisy AI.vi"("Waveguide Cluster"=T15 {"I+"=0, "I-"=1, "V+"=2, "V-"=3, "Vsg"=4}, "error in (no error)"=w1174, "Instrument.DAQ in"=w1176) -> ("error out"=w1175:errorcluster, "Instrument.DAQ out"=w1171:refnum<class "Instrument.DAQ.lvclass">)  [unwired: 5 in, 2 out]
            n549 = Bundle By Name(cluster=w1172, "SMO"=w1171) -> (w1173:T19)
            n550 = call <vilib>:"Add State(s) to Queue__jki_lib_state_machine.vi"("State(s) in (\"\")"=w1179) -> ("States Out"=w1178:string)  [unwired: 14 in]
          }
          frame "DSP: Phase" {
            # "unused"
            n551 = Unbundle By Name(w1195) -> ("SMO"=w1188:refnum<class "Instrument.DAQ.lvclass">, "Results"=w1187:T18)
            n552 = call "Set REF Phase to Zero.vi"("error in (no error)"=w1192, "Reset Phase"="Reset REF", "Instrument.DAQ"=w1188) -> ("error out"=w1182:errorcluster, "Instrument.DAQ out"=w1184:refnum<class "Instrument.DAQ.lvclass">)  [unwired: 7 in]
            n553 = case shown="True" "Auto Phase" {
              tunnel: w1184 -> [w1201 w1205]
              tunnel: [w1201 w1204] -> w1183
              tunnel: w1182 -> [w1200 w1203]
              tunnel: [w1200 w1202] -> w1181
              frame False {
              }
              frame True {
                n554 = call "PLL.vi"("error in (no error)"=w1203, "Instrument.DAQ in"=w1205) -> ("error out"=w1202:errorcluster, "Instrument.DAQ out"=w1204:refnum<class "Instrument.DAQ.lvclass">)  [unwired: 6 in, 2 out]
              }
            }
            n555 = call "Calibrate Phase.vi"("error in (no error)"=w1181, "Boolean"="Calibrate Phase", "Results"=w1187, "Instrument.DAQ in"=w1183) -> ("error out"=w1190:errorcluster, "Instrument.DAQ out"=w1189:refnum<class "Instrument.DAQ.lvclass">)  [unwired: 6 in]
            n556 = flat-sequence {
              tunnel: w1190 -> [w1207]
              tunnel: [w1207] -> w1186
              frame #0 {
                n557 = local write "Calibrate Phase"(FALSE) -> ()
              }
            }
            n558 = call "Replace AO and REF Ch.vi"("error in (no error)"=w1186, "Instrument.DAQ (NEW)"=w1189, "Instrument.DAQ (OLD)"=w1188) -> ("error out"=w1185:errorcluster, "Instrument.DAQ out"=w1193:refnum<class "Instrument.DAQ.lvclass">)  [unwired: 7 in]
            n559 = Bundle By Name(cluster=w1195, "SMO"=w1193) -> (w1194:T19)
            n560 = call <vilib>:"Add State(s) to Queue__jki_lib_state_machine.vi"("State(s) in (\"\")"=w1199) -> ("States Out"=w1198:string)  [unwired: 14 in]
          }
          frame "DSP: Filter" {
            # "publish waveforms"
            # "does not put filtered waveforms on class wire"
            n561 = Unbundle By Name(w1226) -> ("SMO"=w1224:refnum<class "Instrument.DAQ.lvclass">)
            n562 = call "Subtract DAQ Offset.vi"("error in (no error)"=w1223, "Instrument.DAQ"=w1224) -> ("error out"=w1216:errorcluster, "Instrument.DAQ out"=w1210:refnum<class "Instrument.DAQ.lvclass">)  [unwired: 8 in]
            n563 = Unbundle By Name(w1210) -> ("AO"=w1221:waveform(dbl)[], "AI"=w1209:waveform(dbl)[], "REF_X"=w1219:waveform(dbl)[], "REF_Y"=w1218:waveform(dbl)[], "X"=w1220:waveform(dbl)[], "Y"=w1212:waveform(dbl)[])
            n564 = call "Prefilter.vi"("error in (no error)"=w1216, "Waveforms in"=w1209, "Instrument.DAQ in"=w1210) -> ("error out"=w1214:errorcluster, "Waveforms out"=w1208:waveform(dbl)[], "Instrument.DAQ out"=w1215:refnum<class "Instrument.DAQ.lvclass">)  [unwired: 6 in]
            n565 = Bundle By Name(cluster=T16 {"AO"=[], "AI"=[], "REF_X"=[], "REF_Y"=[], "X"=[], "Y"=[]} ("Waveforms"), "AO"=w1221, "AI"=w1208, "REF_X"=w1219, "REF_Y"=w1218, "X"=w1220, "Y"=w1212) -> (w1217:T16)
            n566 = call "DAQ.getWaveforms.vi"("error in (no error)"=w1214, "Waveforms"=w1217, "Instrument.DAQ"=w1215) -> ("error out"=w1213:errorcluster, "Instrument.DAQ"=w1211:refnum<class "Instrument.DAQ.lvclass">)  [unwired: 7 in]
            n567 = Bundle By Name(cluster=w1226, "SMO"=w1211) -> (w1225:T19)
            n568 = call <vilib>:"Add State(s) to Queue__jki_lib_state_machine.vi"("State(s) in (\"\")"=w1229) -> ("States Out"=w1228:string)  [unwired: 14 in]
          }
          frame "DSP: Lockin" {
            n569 = Unbundle By Name(w1243) -> ("SMO"=w1233:refnum<class "Instrument.DAQ.lvclass">)
            n570 = flat-sequence {
              tunnel: [w1259] -> w1238
              tunnel: w1232 -> [w1258]
              tunnel: [w1258] -> w1241
              frame #0 {
                n571 = call <vilib>:"High Resolution Relative Seconds.vi"() -> ("relative seconds"=w1259:dbl)
              }
            }
            n572 = call "Lockin.Engine.vi"("error in (no error)"=w1241, "Instrument.DAQ"=w1233) -> ("error out"=w1239:errorcluster, "Results (X,Y,R,Theta,Mean)"=w1235:T18, "Instrument.DAQ out"=w1234:refnum<class "Instrument.DAQ.lvclass">, "Continue DSP?"=w1231:bool)  [unwired: 5 in, 1 out]
            n573 = flat-sequence {
              tunnel: [w1257] -> w1240
              tunnel: w1239 -> [w1256]
              tunnel: [w1256] -> w1230
              frame #0 {
                n574 = call <vilib>:"High Resolution Relative Seconds.vi"() -> ("relative seconds"=w1257:dbl)
              }
            }
            n575 = case shown="True" w1231 {
              tunnel: w1243 -> [w1248 w1255]
              tunnel: [w1248 w1254] -> w1242
              tunnel: [w1247 w1252] -> w1237
              tunnel: w1235 -> [_ w1251]
              tunnel: w1234 -> [_ w1250]
              tunnel: w1230 -> [w1247 w1249]
              frame False {
              }
              frame True {
                # "publish Results"
                n576 = call "DAQ.getResults.vi"("error in (no error)"=w1249, "Results"=w1251, "Instrument.DAQ"=w1250) -> ("error out"=w1252:errorcluster, "Instrument.DAQ out"=w1253:refnum<class "Instrument.DAQ.lvclass">)  [unwired: 7 in]
                n577 = Bundle By Name(cluster=w1255, "SMO"=w1253, "Results"=w1251) -> (w1254:T19)
              }
            }
            n578 = Subtract(x=w1240, y=w1238) -> (x-y=→"DSP (s)" →"DSP Chart":dbl)
            n579 = call <vilib>:"Add State(s) to Queue__jki_lib_state_machine.vi"("State(s) in (\"\")"=w1246) -> ("States Out"=w1245:string)  [unwired: 14 in]
          }
          frame "DSP: Route" {
            n580 = Unbundle By Name(w1260) -> ()  [unwired: 1 out]
            n581 = call <vilib>:"Add State(s) to Queue__jki_lib_state_machine.vi"("State(s) in (\"\")"=w1264) -> ("States Out"=w1263:string)  [unwired: 14 in]
          }
          frame "DSP: Measure DAQ Offset" {
            w1278 = FALSE ("measureOffset")
            # "this is only a set method"
            # "multiply by gain to get signal at ADC"
            # "AO/AI divides by gain"
            # "This state happens before any offset is subtracted\n(so no need to subtract any offsets first...)"
            # "reset indicator after measuring"
            n582 = Unbundle By Name(w1281) -> ("SMO"=w1275:refnum<class "Instrument.DAQ.lvclass">)
            n583 = Unbundle By Name(w1275) -> ("AI"=w1265:waveform(dbl)[])
            n584 = call "Multiply Waveform by Input Gain.vi"("error in (no error)"=w1266, "WFM in"=w1265, "Instrument.DAQ"=w1275) -> ("error out"=w1274:errorcluster, "WFM out"=w1272:waveform(dbl)[], "Instrument.DAQ out"=w1276:refnum<class "Instrument.DAQ.lvclass">)  [unwired: 6 in]
            n585 = call-poly <vilib>:"Basic Averaged DC-RMS.vi"("reset"=TRUE, "error in (no error)"=w1274, "signals in"=w1272) -> ("error out"=w1277:errorcluster, "DC values"=w1271:dbl[])  [unwired: 5 in, 2 out]
            n586 = call "Set DAQ Offset.vi"("error in (no error)"=w1277, "Offsets"=w1271, "Instrument.DAQ"=w1276) -> ("error out"=w1268:errorcluster, "Instrument.DAQ out"=w1270:refnum<class "Instrument.DAQ.lvclass">)  [unwired: 7 in]
            n587 = Unbundle By Name(w1270) -> ("Offset_AI"=w1269:T69)
            n588 = call "DAQ.getInputOffset.vi"("error in (no error)"=w1268, "Input Offset"=w1269, "Instrument.DAQ"=w1270) -> ("error out"=w1267:errorcluster, "Instrument.DAQ out"=w1273:refnum<class "Instrument.DAQ.lvclass">)  [unwired: 7 in]
            n589 = Bundle By Name(cluster=w1281, "SMO"=w1273, "Measure Offset"=w1278) -> (w1280:T19)
            n590 = local write "Measure Offset"(w1278) -> ()
            n591 = call <vilib>:"Add State(s) to Queue__jki_lib_state_machine.vi"("State(s) in (\"\")"=w1284) -> ("States Out"=w1283:string)  [unwired: 14 in]
          }
          frame "DSP: Zero DAQ Offset" {
            # "reset indicator after zeroing"
            n592 = Unbundle By Name(w1297) -> ("SMO"=w1295:refnum<class "Instrument.DAQ.lvclass">)
            n593 = Unbundle By Name(w1295) -> ("AI"=w1292:waveform(dbl)[])
            n594 = Array Size(array=w1292) -> (size(s)=w1293:i32)
            n595 = Initialize Array(0.0, w1293) -> (w1285:dbl[])
            n596 = call "Set DAQ Offset.vi"("error in (no error)"=w1294, "Offsets"=w1285, "Instrument.DAQ"=w1295) -> ("error out"=w1289:errorcluster, "Instrument.DAQ out"=w1287:refnum<class "Instrument.DAQ.lvclass">)  [unwired: 7 in]
            n597 = Unbundle By Name(w1287) -> ("Offset_AI"=w1290:T69)
            n598 = call "DAQ.getInputOffset.vi"("error in (no error)"=w1289, "Input Offset"=w1290, "Instrument.DAQ"=w1287) -> ("error out"=w1288:errorcluster, "Instrument.DAQ out"=w1286:refnum<class "Instrument.DAQ.lvclass">)  [unwired: 7 in]
            n599 = local write "Zero Offset"(FALSE ("measureOffset")) -> ()
            n600 = Bundle By Name(cluster=w1297, "SMO"=w1286) -> (w1296:T19)
            n601 = call <vilib>:"Add State(s) to Queue__jki_lib_state_machine.vi"("State(s) in (\"\")"=w1301) -> ("States Out"=w1300:string)  [unwired: 14 in]
          }
          frame "---------- Sweep ----------" {
            n602 = call <vilib>:"Add State(s) to Queue__jki_lib_state_machine.vi"("State(s) in (\"\")"=w1306) -> ("States Out"=w1305:string)  [unwired: 14 in]
          }
          frame "Sweep: Initialize" {
            n603 = Get Date/Time In Seconds() -> (seconds since 1Jan1904=w1309:timestamp)
            n604 = To Double Precision Float(number=w1309) -> (double precision float=→"Sweep Start":dbl)
            n605 = call <vilib>:"Add State(s) to Queue__jki_lib_state_machine.vi"("State(s) in (\"\")"=w1313) -> ("States Out"=w1312:string)  [unwired: 14 in]
          }
          frame "----------  Generator ----------" {
            n606 = call <vilib>:"Add State(s) to Queue__jki_lib_state_machine.vi"("State(s) in (\"\")"=w1318) -> ("States Out"=w1317:string)  [unwired: 14 in]
          }
          frame "Generator: Start" {
            n607 = Unbundle By Name(w1324) -> ("SMO"=w1323:refnum<class "Instrument.DAQ.lvclass">)
            n608 = Unbundle By Name(w1323) -> ("Generator"=w1322:refnum<class "Generator.lvclass">)
            n609 = call "setCommand.vi"("error in (no error)"=w1320, "command"=Generator.Command--enum."start", "Generator in"=w1322) -> ("error out"=w1321:errorcluster)  [unwired: 7 in, 1 out]
            n610 = call <vilib>:"Add State(s) to Queue__jki_lib_state_machine.vi"("State(s) in (\"\")"=w1327) -> ("States Out"=w1326:string)  [unwired: 14 in]
          }
          frame "Generator: Start Sweep" {
            n611 = Unbundle By Name(w1333) -> ("SMO"=w1332:refnum<class "Instrument.DAQ.lvclass">)
            n612 = Unbundle By Name(w1332) -> ("Generator"=w1331:refnum<class "Generator.lvclass">)
            n613 = call "setCommand.vi"("error in (no error)"=w1329, "command"=Generator.Command--enum."start sweep", "Generator in"=w1331) -> ("error out"=w1330:errorcluster)  [unwired: 7 in, 1 out]
            n614 = call <vilib>:"Add State(s) to Queue__jki_lib_state_machine.vi"("State(s) in (\"\")"=w1336) -> ("States Out"=w1335:string)  [unwired: 14 in]
          }
          frame "Generator: Stop" {
            n615 = Unbundle By Name(w1342) -> ("SMO"=w1341:refnum<class "Instrument.DAQ.lvclass">)
            n616 = Unbundle By Name(w1341) -> ("Generator"=w1340:refnum<class "Generator.lvclass">)
            n617 = call "setCommand.vi"("error in (no error)"=w1338, "command"=Generator.Command--enum."stop", "Generator in"=w1340) -> ("error out"=w1339:errorcluster)  [unwired: 7 in, 1 out]
            n618 = call <vilib>:"Add State(s) to Queue__jki_lib_state_machine.vi"("State(s) in (\"\")"=w1345) -> ("States Out"=w1344:string)  [unwired: 14 in]
          }
          frame "Generator: Stop Sweep" {
            n619 = Unbundle By Name(w1351) -> ("SMO"=w1350:refnum<class "Instrument.DAQ.lvclass">)
            n620 = Unbundle By Name(w1350) -> ("Generator"=w1349:refnum<class "Generator.lvclass">)
            n621 = call "setCommand.vi"("error in (no error)"=w1347, "command"=Generator.Command--enum."stop sweep", "Generator in"=w1349) -> ("error out"=w1348:errorcluster)  [unwired: 7 in, 1 out]
            n622 = call <vilib>:"Add State(s) to Queue__jki_lib_state_machine.vi"("State(s) in (\"\")"=w1354) -> ("States Out"=w1353:string)  [unwired: 14 in]
          }
        }
      }
    }
    frame Error {
    }
  }
  n623 = call-parent "Process.vi"("error in"=w5, "SMO"=w4) -> ("error out"=w2:errorcluster, "SMO out"=→"Instrument.DAQ out":refnum<class "Instrument.DAQ.lvclass">)  [unwired: 8 in]
  n624 = Merge Errors(w2, w1) -> (→"error out":errorcluster)
